vi "MAIN_8.1.vi"() -> ()   [LabVIEW 2015]
doc: "Use this template to build a producer/consumer design pattern with events to produce queue items. Use this design pattern instead of the User Interface Event Handler pattern for user interfaces when you want to execute code asynchronously in response to an event without slowing the user interface responsiveness."
uses:
  State_machine_enum.ctl
  display2.ctl
  User_buttons_enum.ctl
  <vilib>/Analysis/baseanly.llb/Mean (DBL).vi
  <vilib>/DAQmx/read.llb/DAQmx Read (Analog 2D DBL NChan NSamp).vi
  Global 1_diag.vi
  <vilib>/Waveform/WDTFileIO.llb/Export Waveforms To Spreadsheet File (1D).vi
  <vilib>/Utility/file.llb/Write To Spreadsheet File (DBL).vi
  <vilib>/DAQmx/create/channels.llb/DAQmx Create Channel (AI-Voltage-Basic).vi
  <vilib>/DAQmx/configure/timing.llb/DAQmx Timing (Sample Clock).vi
  <vilib>/DAQmx/miscellaneous.llb/DAQmx Fill In Error Info.vi
  <vilib>/express/express arith-compare/Formula/XNode/ExpressFormulaBlockNode.xnode
  <vilib>/Analysis/NI_AALBase.lvlib
  <resource>/objmgr/daqmx.rc
panel:
  out "2f Spectrum array":dbl[](array[numeric])
  out "x/y":dbl=0.002005684477504462
  in  "Motor Voltage (V) 2":dbl=1.0 min=0.0 max=9.0
  in  "Time Resolved":bool=TRUE
  in  "Start time":timestamp=timestamp(-9593251199.274853 s since 1904-01-01)
  in  "Timer Start":bool
  out "path":path=path "C:/Users/Adam/Desktop/Diag_Prog_v9/temp.txt"
  in  "Stabilization Time (s)":dbl min=0.0 max=2.0
  out "LD error array disc":dbl[](array[numeric])
  out "LD array disc":dbl[](array[numeric])
  out "result":bool=TRUE
  out "dt":dbl=0.001
  out "dLD_RMS":dbl=-0.0
  out "error out":errorcluster
  out "Unbalanced?":bool
  out "Signal Balance":bool
  out "DC Voltage (V) 2":dbl(knob)=0.000879695520089483 scale=0.0..10.0
  out "2f Frequency (Hz)":dbl(knob)=512.4961246512186 scale=0.0..150.0
  in  "Voltage Divider (10)":bool
  out "Actual Task":string="Processing signal"
  out "Motor Voltage (V)":dbl=1.0
  in  "Initial Voltage (V)":dbl=0.35 min=0.0 max=9.0
  in  "Final Voltage (V)":dbl=0.8 min=0.0 max=2.0
  in  "Voltage Step (V)":dbl=0.065 min=0.0 max=1000.0
  in  "Motor Stabilization Time (s)":dbl(knob)=10.0 step=0.001 scale=0.0..30.0
  out "Initial Voltage (V) 2":dbl=1.0 min=0.0 max=9.0
  in  "Final Voltage (V) 2":dbl=1.4 min=0.0 max=2.0
  in  "Voltage Step (V) 2":dbl=0.1 min=0.0 max=1000.0
  in  "Comment (sample no)":string
  in  "Stop Measurement":bool
  in  "Start Measurement Button":bool
  out "Measurement File":path=path "C:/Users/Adam/Desktop/Diag_Prog_v9/testt"
  in  "New File":bool
  out "Reset?":bool=TRUE
  out "Actual State":T1=enum."Process"
  in  "Tab Control":T2(tab)=enum."Options"
  out "Measured Points":T3 format="%0.3f"
  out "Ready?":bool
  out "Ready?":string="Ready?"
  out "Motor":bool=TRUE
  out "Motor":string="Motor: OK"
  out "Quick Status 5":string
  out "Down 2":bool
  out "Up 2":bool
  out "Oscilloscope 2":waveform(dbl)[](graph)=[{"t0"=timestamp(0 s since 1904-01-01), "dt"=0.002, "Y"=array[500 elements]}, {"t0"=timestamp(0 s since 1904-01-01), "dt"=0.002, "Y"=array[500 elements]}]
  out "Signal Balance":bool=TRUE
  out "Laser Noise":bool=TRUE
  out "Signal Balance":string="Signal Balance: OK"
  out "Laser Noise":string="Laser Noise: OK"
  in  "Run Quick Diagnostics":bool
  out "Laser Intensity":bool=TRUE
  out "Laser Intensity":string="Laser Intensity: OK"
  out "Delta":T3 format="%0.3f"
  out "Quick Diagnosis":string="?"
  out "Infected?":bool
  out "Detected Signal (mV/V)":T3 format="%0.3f"
  in  "Measure":bool
  out "Signal Spectrum (mVrms/Vdc) 2":cluster{"f0":dbl, "df":dbl, "magnitude":dbl[]}(graph)={"f0"=0.0, "df"=0.05, "magnitude"=[]}
  in  "QuickDiag":bool
  in  "Convert mld":bool
  in  "Convert parasiteno":bool
  in  "Convert parasitemia":bool
  in  "Convert cc":bool
  out "MLD (mV/V)":dbl=3.234067345901155 format="%#_3g"
  out "SA 1f (mv/V)":dbl=2.8989130211772483
  out "Lock_in (mV/V)":dbl
  out "dLock_in (mV/V)":dbl
  out "dMLD (mV/V)":dbl=1.4958145805121073 format="%#_3g"
  out "Phase (deg)":dbl=0.5117629371467104 format="%0.2f"
  out "Phase  dev (deg)":dbl=-1.4797919911802346 format="%0.2f"
  out "SA 2f (mv/V)":dbl=4.7886484733621755
  out "MLD Amplitude (mV/V)":cluster{dbl[], dbl[]}(graph)
  in  "dT/T (%)":dbl
  in  "Dilution":dbl=20.0
  in  "Undiluted cc.\n (ng/ml)":dbl
  in  "Undiluted \nParasitemia (%)":dbl format="%#_6f"
  in  "Parasites/ul\nof Blood":dbl
  in  "Convert dT":bool
  in  "MLD (mV/V)":dbl
  out "DC (V)":cluster{dbl[], dbl[]}(graph)
  out "MLD Phase":cluster{dbl[], dbl[]}(graph)
  out "Down":bool
  out "Up":bool
  out "2f Frequency (Hz)":T3=23.056300268096514 format="%0.3f"
  out "1f SA (mV/V)":T3=153.49895465158366 format="%0.3f"
  out "MLD Sim. LIA (mV/V)":T3=nan format="%0.3f"
  out "MLD SA (mV/V)":T3=37.38207236557522 format="%0.3f"
  in  "Start Scope":bool
  in  "Constant Motor Voltage":dbl=1.0 min=0.0 max=3.0
  in  "Refresh in (s)":i8=10
  in  "stop":bool
  in  "AC?":bool
  out "levelB":dbl=0.1 format="%#_2g"
  out "levelA":dbl format="%#_3g"
  in  "V/div B":dbl(knob)=0.2 scale=10.0..0.01 scale format="%#_3g"
  in  "level B":dbl(slide)=0.4 scale=-1.0..1.0 scale format="%#_3g"
  in  "level A":dbl(slide) scale=-1.0..1.0 scale format="%#_3g"
  in  "V/div A":dbl(knob)=0.05 scale=10.0..0.01 scale format="%#.3f"
  out "Oscilloscope":waveform(dbl)[](graph)=[{"t0"=timestamp(0 s since 1904-01-01), "dt"=0.0025, "Y"=array[375 elements]}, {"t0"=timestamp(0 s since 1904-01-01), "dt"=0.0025, "Y"=array[375 elements]}]
  in  "Sensitivity":T4(ring)
  in  "samples per channel":i32=1000
  in  "rate":dbl=1000.0 format="%0.2f"
  out "Spectrum (mVRMS/Vdc)":cluster{"f0":dbl, "df":dbl, "magnitude":dbl[]}(graph)={"f0"=0.0, "df"=1.0, "magnitude"=[1338.0484216778725, 891.4717650116102, 143.2192215595614, 172.79898091711885, 95.50453001628563, 113.23096269717587, 159.9728459536367, 142.17510842649094, 23.555096842939967, 172.4586840116519, 233.3391086271948, 153.49895465158366, 59.303017218056304, 51.41913744169332, 87.60985790792097, 89.15548748523767, 102.41083253503767, 116.69415211742178, 102.04780407888852, 98.07941394008398, 62.015801498942174, 57.365633541451224, 37.38207236557522, 140.01194138717574, 88.85968438008766, 51.8911573784031, 96.44625566359282, 102.80626369349147, 154.32416325374467, 152.72565881880075, 63.97627104136422, 44.061183722532256, 24.299532372372934, 66.51944362511281, 119.45636901763923, 79.60274206424093, 126.46507446936278, 115.56735495111872, 86.92439368676867, 42.47483057858276, 45.987972767001125, 82.38613913097223, 57.14235729256332, 24.715704736492583, 91.95786457200892, 229.45656360476565, 301.7932887816684, 181.94479488218664, 9.707170408716356, 79.16705422107816, 32.4671901662433, 34.994674897672475, 45.603676560961965, 81.17087782317107, 123.48392300390853, 125.53549820312338, 197.71297955832767, 51.56670220175255, 139.4897349387358, 136.00021553543283, 49.84751230386803, 106.388211919061, 128.21302631973177, 179.83380975700697, 238.686425101159, 204.64888147263136, 159.4400865495827, 88.9566203515302, 50.82386237011203, 47.10090178269198, 31.249556983451996, 155.07366739734923, 197.20488460315576, 181.86491698592144, 122.60135896300172, 15.723508058553668, 47.32988919426525, 91.09235604990127, 70.08764782926058, 71.11042986773145, 167.58334514547386, 157.0684001711449, 85.4088975978964, 165.68125229281705, 108.34787076535925, 58.32465184772515, 102.85811162079386, 88.031264754637, 35.99088343784742, 74.99228300753498, 59.59436041355427, 109.74543517855098, 239.92689639368845, 195.22681808589817, 153.93792803433803, 171.35120542643082, 103.04216715301814, 144.22424620891795, 33.236928017526, 33.6474288996255, 71.18496484217899, 175.10446025244616, 221.24997378317522, 114.75466832528755, 52.3833439055373, 114.90211538243959, 94.87498722211751, 82.82924122532899, 124.12586199482064, 107.6258638888207, 78.5024563400891, 92.06245924719637, 16.228987466475928, 84.84217000760313, 88.76503911599063, 114.25618103440272, 155.27289903749065, 116.20062823456668, 61.96139303164934, 214.19314697712042, 248.12058486418763, 215.9112937618697, 145.04293815290015, 142.16464369485132, 169.7377761460246, 83.55657324380019, 74.4879617799582, 39.81106304135121, 152.2410798694005, 176.4879867987291, 110.01229615691923, 89.83888006443468, 195.69702436303007, 166.19892376632072, 55.02836867851484, 113.06515146784245, 221.3685360221306, 181.10055208661387, 262.0371181638539, 185.73443857709046, 93.90961856721144, 84.54783744027858, 24.449872475327695, 95.3789149136639, 140.24246950513043, 143.73337464437884, 33.58378655631947, 62.839362697344995, 57.47449635929643, 139.96968907631262, 167.0231838520772, 135.6723918020847, 124.14523269479409, 111.37946391963057, 195.70470757666732, 192.9947832776428, 93.91006382282066, 121.56931305302999, 113.63589006917633, 42.92804035457153, 141.48803985115433, 165.5507518379778, 121.34962379960878, 143.04362518480343, 22.72432951654588, 183.17549468524615, 152.95042171438013, 195.3079831947777, 131.83171839040367, 30.49881104219535, 8.46043248589554, 141.40803256070282, 223.72992955634092, 132.30059550265176, 54.60897309407436, 84.56504745319246, 125.72411835874722, 194.72474433717994, 126.94182365881618, 27.456941187399302, 114.85067679816903, 138.3914927403539, 237.22038521157256, 172.58040690453, 178.93819766022105, 171.11586449112946, 66.32529189912087, 175.61268977844438, 179.0727535154661, 223.71442469320746, 230.52161416220554, 181.0440521026372, 72.70233235363926, 157.99312186800248, 143.29067791998708, 138.45794114882568, 122.15383561979628, 55.90884824057415, 43.2895289444191, 25.99180252149831]}
  out "MLD LIA (mV/V)":dbl=0.0123978
  out "Lockin_freq":dbl=9.4676
  out "DC Voltage (V)":T3=0.000879695520089483 format="%0.3f"
  out "Time Domain Signal":cluster{"xi used":dbl[], "yi":dbl[]}[](graph)
  out "Signal Spectrum (mVrms/Vdc)":cluster{"f0":dbl, "df":dbl, "magnitude":dbl[]}[](graph)
  out "1f 2f Spectral Peaks":T5={"1f (Hz)"=256.112805640282, "U1f (mV/V)"=2.8989130211772483, "2f (Hz)"=512.375618780939, "U2f (mV/V)"=4.7886484733621755}
  out "LockIN Theta (cont/disc)":waveform(dbl)(graph)={"t0"=timestamp(0 s since 1904-01-01), "dt"=0.002, "Y"=[]}
  out "LockIN R (cont/disc)":waveform(dbl)(graph)={"t0"=timestamp(0 s since 1904-01-01), "dt"=0.002, "Y"=[]}
  in  "Pike Removal (StDev)":dbl=3.0
  in  "Lock-in Time (s)":dbl=10.0
  in  "dt (s)":dbl=0.0002
  in  "Resolution (s)":dbl=0.0001
  in  "Averaging time (s)":dbl=1.0 format="%0.2p"
  in  "Cutoff Frequency (Hz)":dbl=500.0
  in  "Rate":dbl=5000.0 caption="Sample Rate (Hz)" format="%0.2f"
  in  "Samples per Channel":i32=100000
  out "Minimum Value":dbl=-1.0 caption="LD min Value (V)" format="%0.2f"
  out "Maximum Value":dbl=1.0 caption="LD max Value (V)" format="%0.2f"
  in  "DC # samples":i32=100
  in  "DC Sampling Rate (Hz)":dbl=100.0
  in  "Dc min":dbl format="%0.2f"
  in  "Dc max":dbl=10.0 format="%0.2f"
  in  "Reference Signal":tag="Dev1/ai3"
  in  "LD Signal":tag="Dev1/ai0" caption="LD Channel"
  in  "DC Voltage DAQ":tag="Dev1/ai1"
  in  "Motor Channel":tag="Dev1/ao1"
  in  "Lock-in-Amplifier VISA":refnum<visa-resource-name>="GPIB0::3::INSTR"
  in  "Second Harmonic":bool
  in  "Lock In":bool
  in  "Continous Lock-in":bool=TRUE
  out "Dc standard deviation":dbl=0.002551891780639937 format="%0.2f"
  out "Dc mean":dbl=0.000879695520089483 format="%0.2f"
  out "dPhase array":dbl[](array[numeric])=[0.7103181848590662, 0.7091849884099535, 0.5117629371467104]
  out "Phase array":dbl[](array[numeric])=[2.6241958943190986, 1.203559524600966, nan, 1.2024263281518537, -0.21594364866805338, nan, -1.4797919911802346]
  out "LD array":dbl[](array[numeric])=[0.8882278113428617, 1.3288564379056984, 3.234067345901155]
  out "Frequency array":dbl[](array[numeric])=[811.3544417222341, 812.123069024086, 812.8874794085821]
  out "LD error array":dbl[](array[numeric])=[0.357199186111431, 0.6995380180896104, 1.4958145805121073]
  out "First?":bool
  out "Stopped":bool
  out "Last Step?":bool
  in  "EXIT":bool
  # "Measurement Settings"
  # "Motor Setup"
  # "OFF"
  # "ON"
  # "Setup"
  # "Status:"
  # "Measurement"
  # "mV/V"
  # "±"
  # "Detected Magneto-Optical Signal:"
  # "Quick Diagnosis Report:"
  # "Measured points:"
  # "Actual Datapoint Values"
  # "Convert quantities"
  # "Physical channels"
  # "Signal Processing Settings"
  # "DC Acquisition Settings"
  # "LD Acquisition Settings"
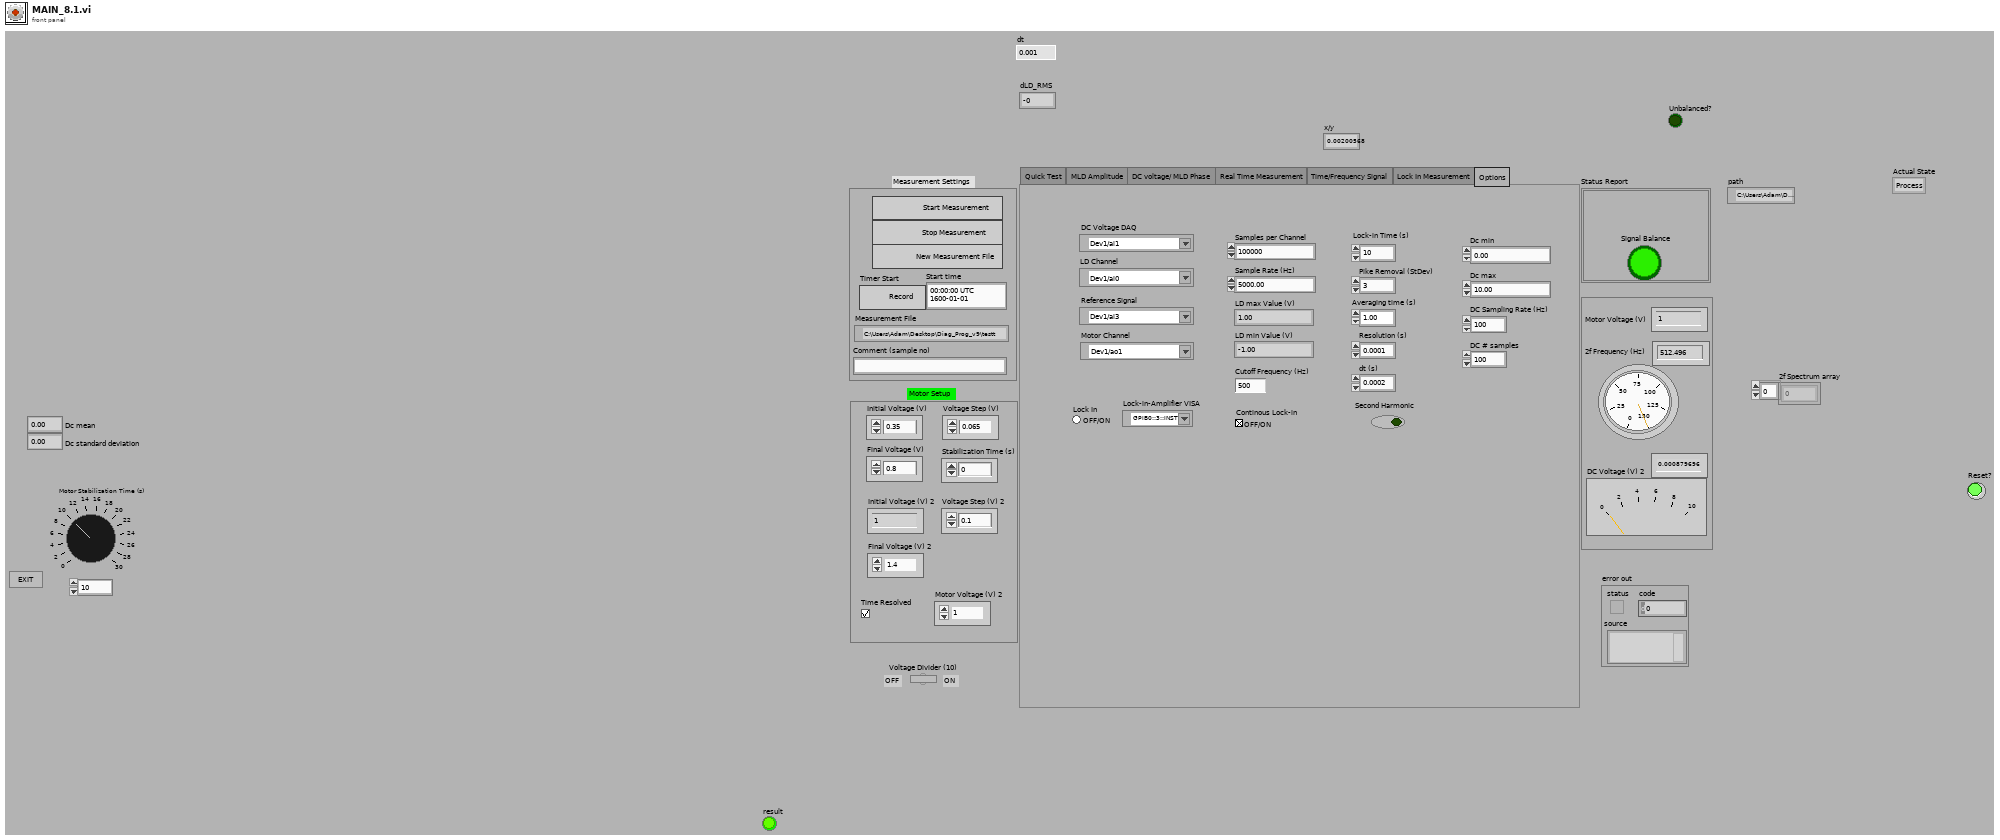
[diagram p1: front panel]
types:
  T1 = typedef "State_machine_enum.ctl" = enum16{"SetMotor", "Stabilize", "Measure", "Process", "Save", "Finished"}
  T2 = enum32{"Quick Test", "MLD Amplitude", "DC voltage/ MLD Phase", "Real Time Measurement", "Time/Frequency Signal", "Lock In Measurement", "Options"}
  T3 = typedef "display2.ctl" = dbl
  T4 = enum16{"-1V..1V", "-1.25V..1.25V", "-2V..2V", "-2.5V..2.5V", "-4V..4V", "-5V..5V", "-10V..10V"}
  T5 = cluster{"1f (Hz)":dbl, "U1f (mV/V)":dbl, "2f (Hz)":dbl, "U2f (mV/V)":dbl}
  T6 = typedef "User_buttons_enum.ctl" = enum16{"start", "stop", "exit", "New", "Scope", "Continue"}
  T7 = enum16{"open", "replace", "create", "open or create", "replace or create", "replace or create with confirmation"}
  T8 = enum8{"Enabled", "Disabled", "Disabled and Grayed Out"}
  T9 = enum16{"Left Button", "Center Button", "Right Button", "Window Close"}
  T10 = cluster{dbl, "1f Ampl (Vrms/Vdc)":dbl, dbl, "2f Ampl (Vrms/Vdc)":dbl}
  T11 = cluster{"MLD":dbl, "dMLD":dbl, "Phase":dbl, "dPhase":dbl}
  T12 = cluster{"Frequency array":dbl[], "LD array":dbl[]}
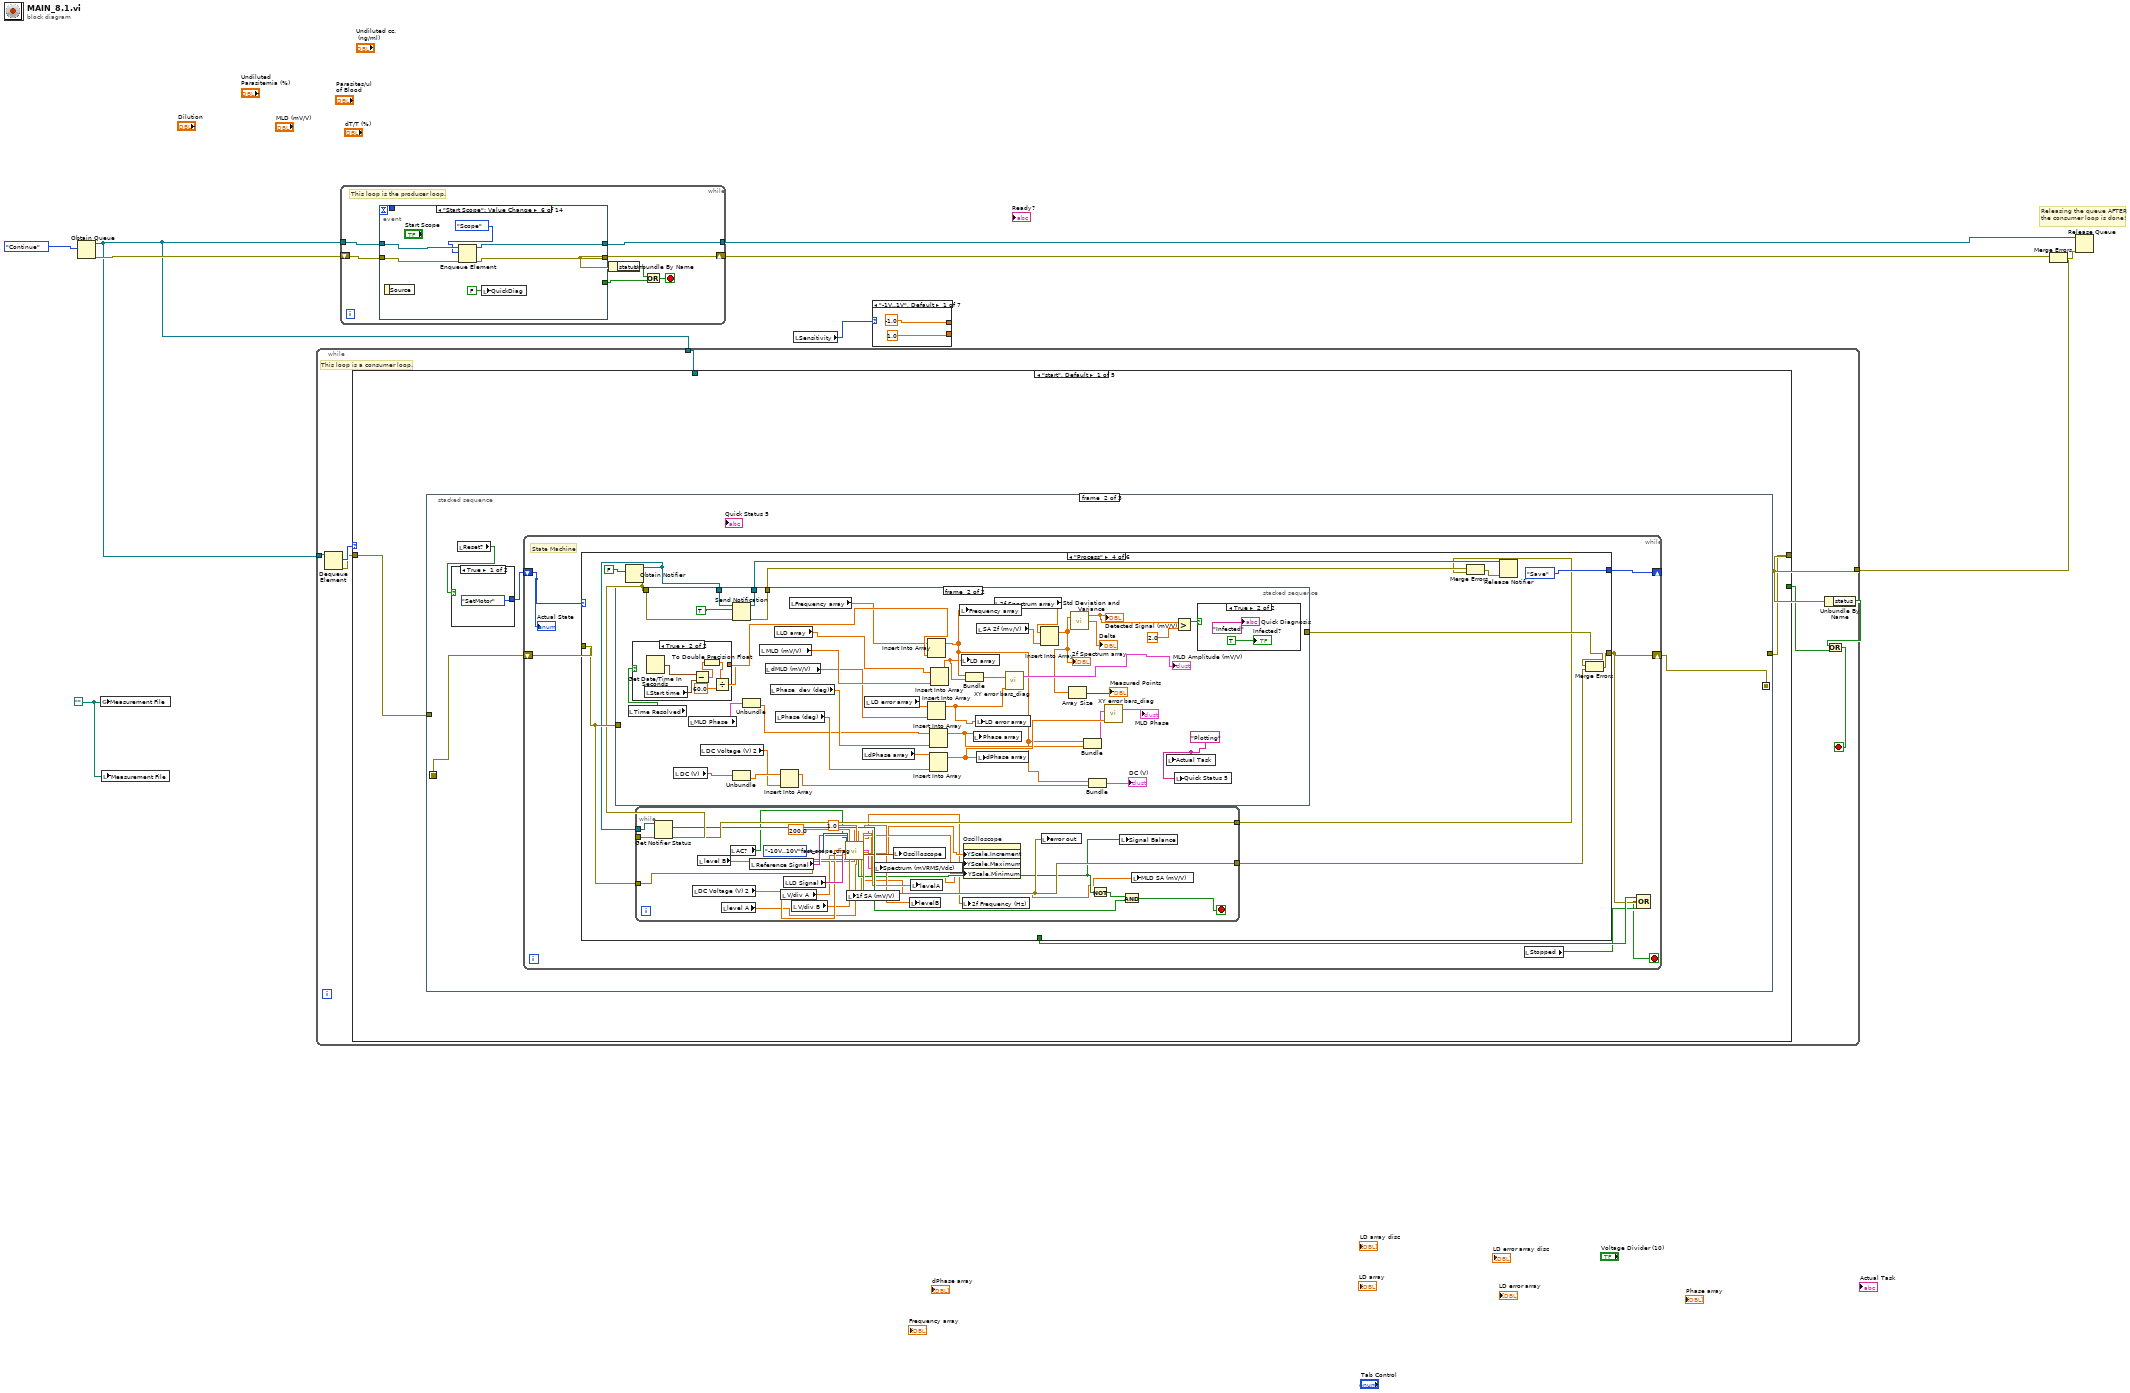
[diagram p0: block diagram]
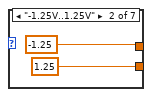
[diagram p2: hidden frame]
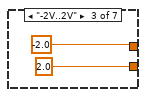
[diagram p3: hidden frame]
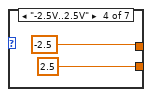
[diagram p4: hidden frame]
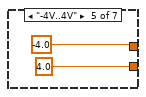
[diagram p5: hidden frame]
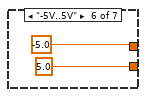
[diagram p6: hidden frame]
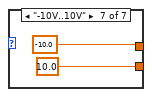
[diagram p7: hidden frame]
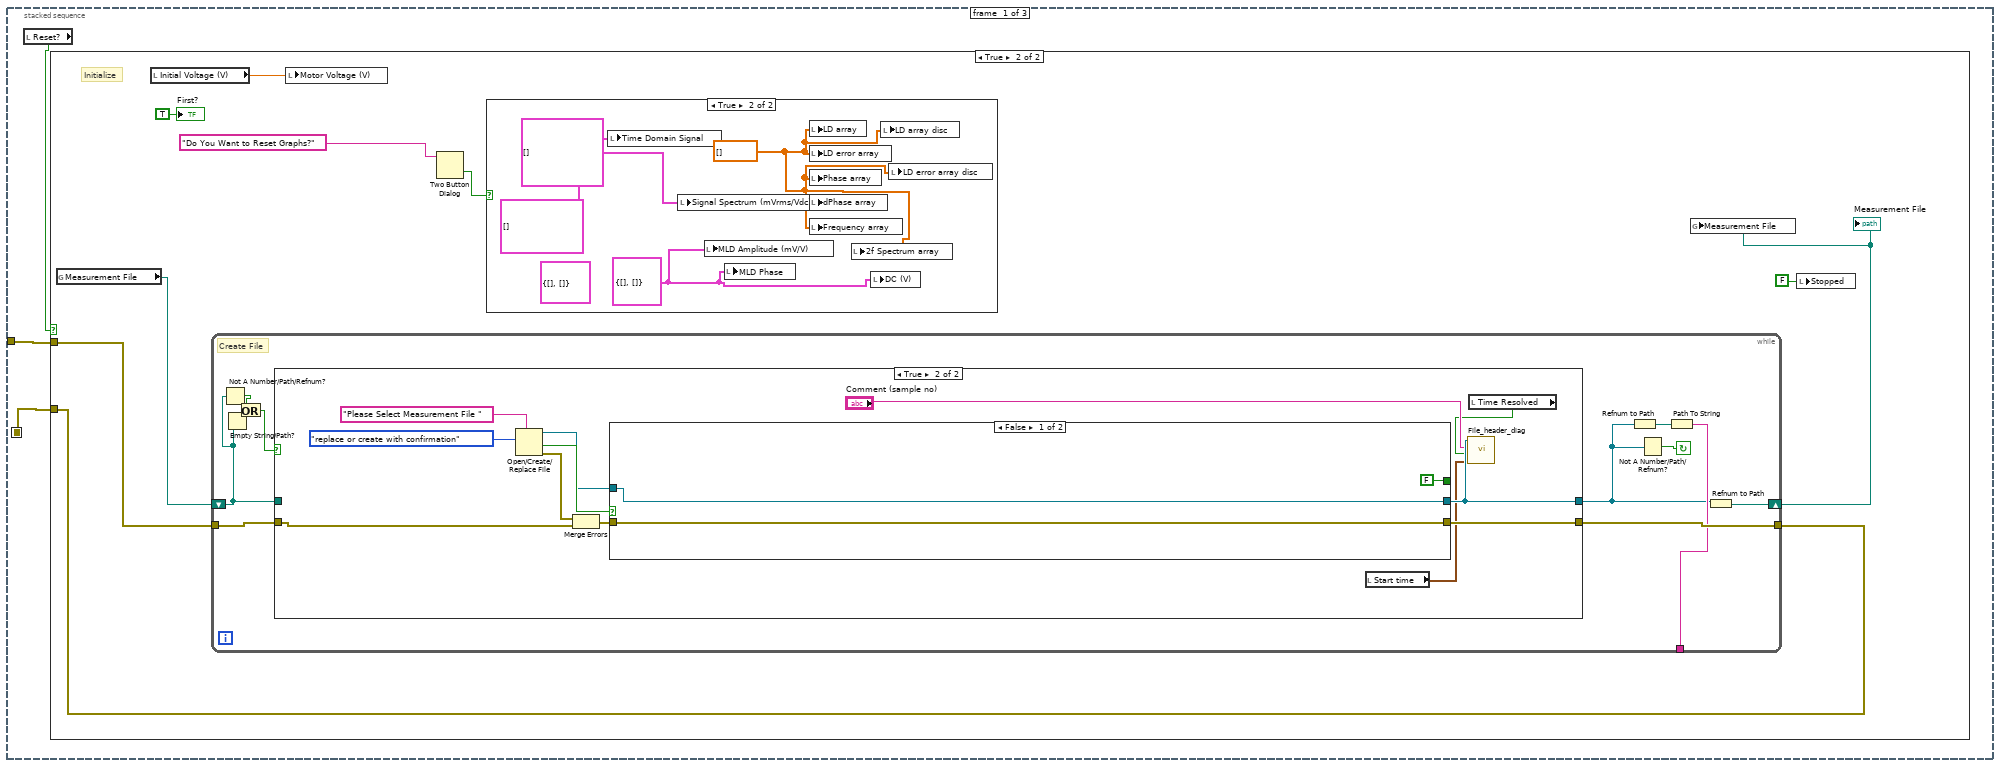
[diagram p8: hidden frame]
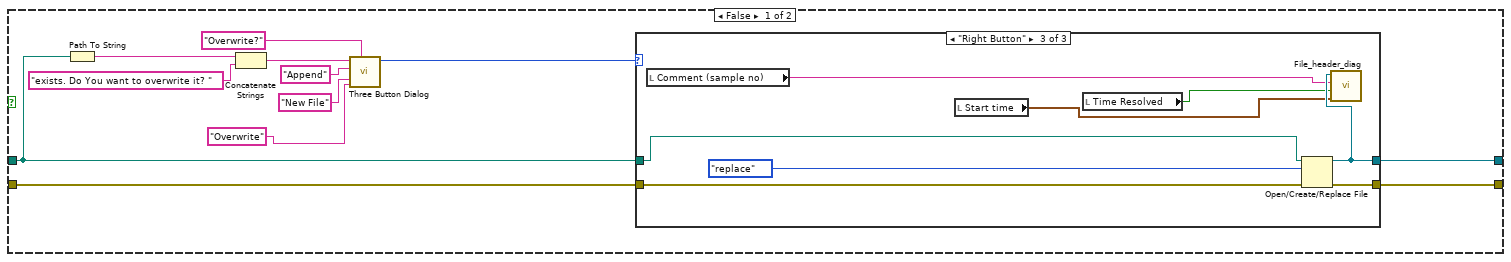
[diagram p10: hidden frame]
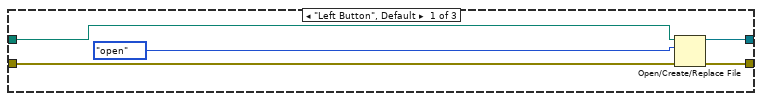
[diagram p11: hidden frame]
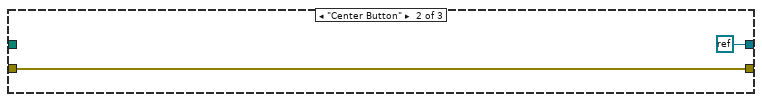
[diagram p12: hidden frame]
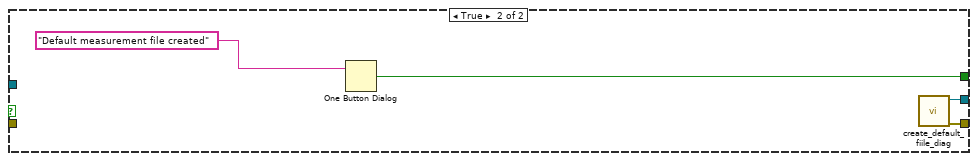
[diagram p13: hidden frame]
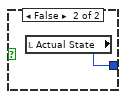
[diagram p15: hidden frame]
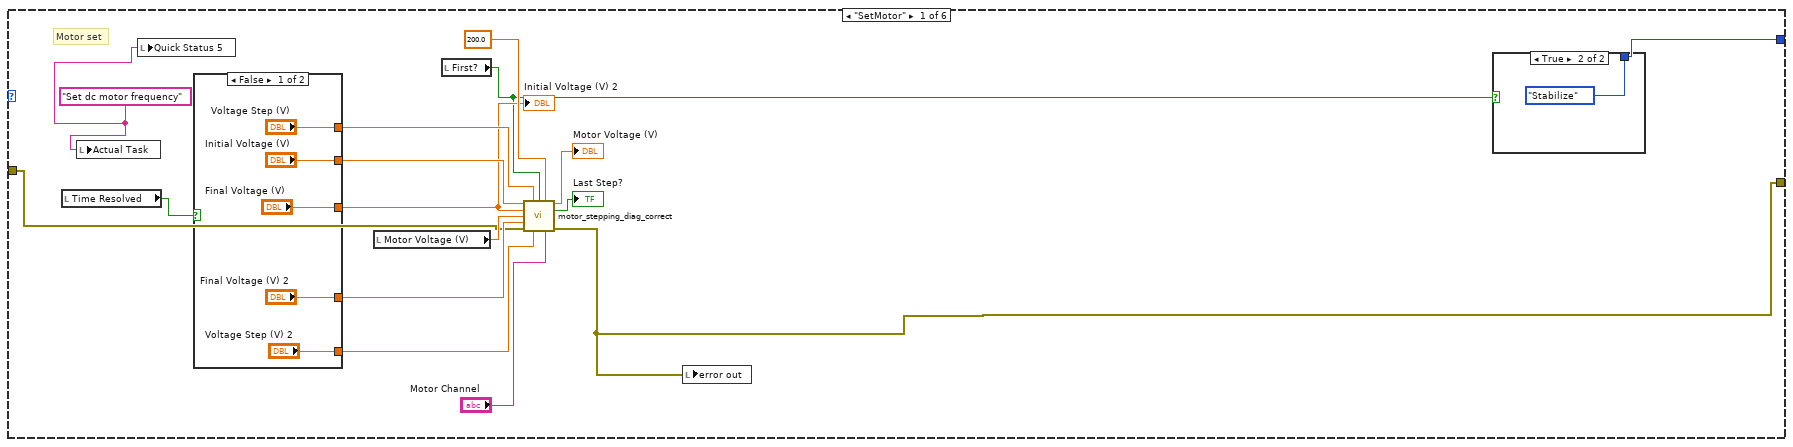
[diagram p16: hidden frame]
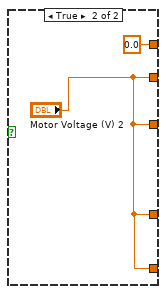
[diagram p17: hidden frame]
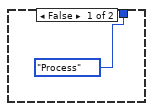
[diagram p18: hidden frame]
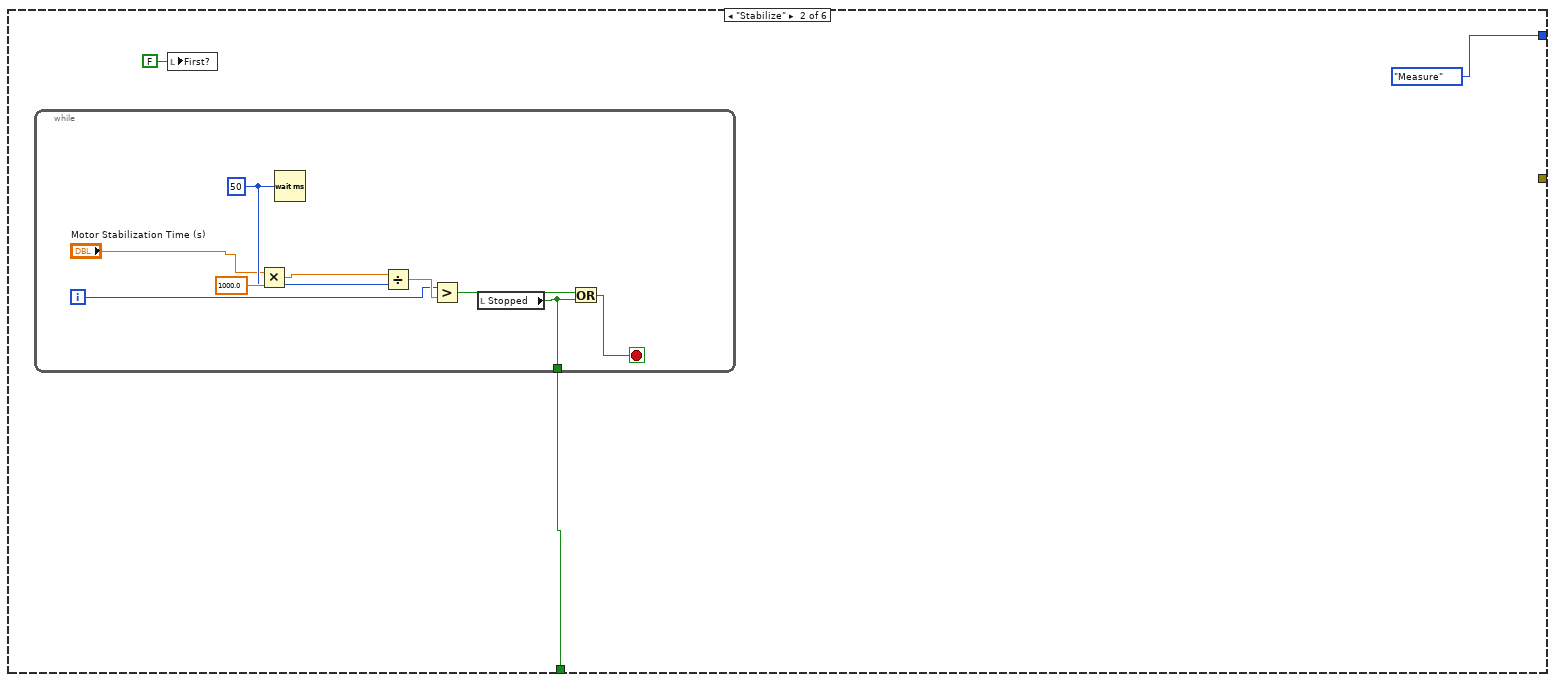
[diagram p19: hidden frame]
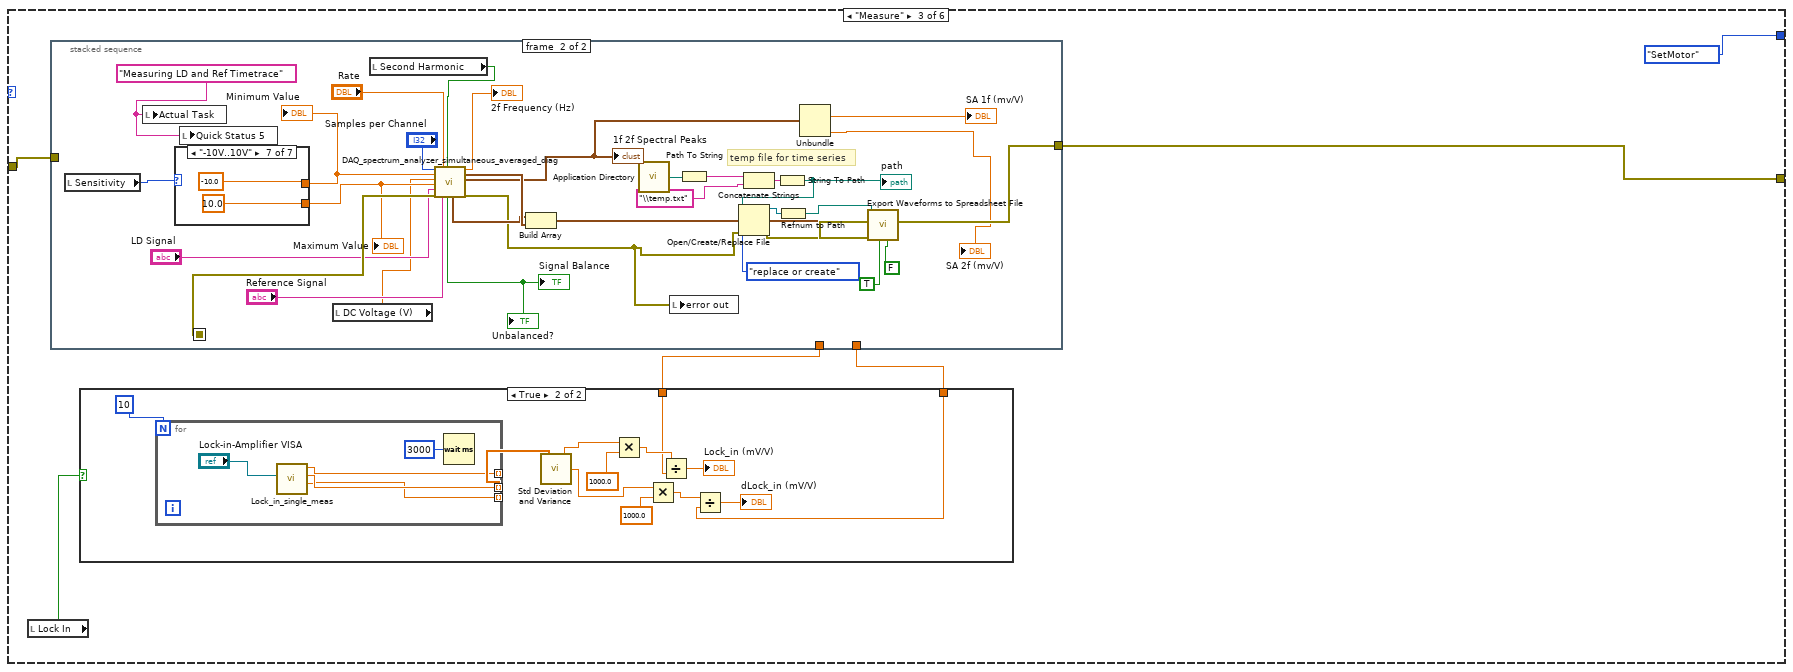
[diagram p20: hidden frame]
diagram:
  w3 = path ""
  # "Releasing the queue AFTER\nthe consumer loop is done!"
  n1 = Obtain Queue(element data type=User_buttons_enum."Continue") -> (queue out=w2:refnum<queue>, error out=w9:errorcluster)  [unwired: 4 in, 1 out]
  n2 = global write "Global 1_diag.vi" "Measurement File"(w3) -> ()
  n3 = local write "Measurement File"(w3) -> ()
  n4 = while {
    tunnel: w2 -> [w17]
    tunnel: [w14] -> w5
    tunnel: w2 -> [w10]
    stop <- w11 stop-if-true
    # "This loop is a consumer loop."
    n5 = Dequeue Element(queue=w17) -> (element=w16:T6, error out=w15:errorcluster)  [unwired: 2 in, 2 out]
    n6 = case shown="\"start\", Default" w16 {
      tunnel: [_ _ TRUE _ _] -> w12
      tunnel: w15 -> [w19 w418 w480 w484 w493]
      tunnel: [w18 w417 w480 w483 w499] -> w14
      tunnel: w10 -> [_ w416 _ _ w485]
      frame "start", Default {
        n7 = stacked-sequence {
          seq-local: [w21 _ _] -> [_ w97 _]
          seq-local: [_ w96 _] -> [_ _ w403]
          tunnel: w19 -> [w22 _ w401]
          tunnel: [_ _ w400] -> w18
          frame #0 {
            n8 = local read "Reset?"() -> (w20:bool)
            n9 = case shown="True" w20 {
              tunnel: w22 -> [w23 w27]
              tunnel: [w23 w25] -> w21
              frame False {
              }
              frame True {
                # "Initialize"
                n10 = global read "Global 1_diag.vi" "Measurement File"() -> (w26:path)
                n11 = local read "Initial Voltage (V)"() -> (w30:dbl)
                n12 = while {
                  tunnel: [w43] -> w25
                  tunnel: w27 -> [w42]
                  shift-right: [w37] -> w24
                  shift-left: w26 -> [w36]
                  tunnel: [w39] -> _
                  stop <- w41 continue-if-true
                  # "Create File"
                  n13 = Not A Number/Path/Refnum?(number/path/refnum=w36) -> (NaN/Path/Refnum?=w35:bool)
                  n14 = Empty String/Path?(string/path=w36) -> (empty?=w34:bool)
                  n15 = Or(x=w35, y=w34) -> (x .or. y?=w33:bool)
                  n16 = case shown="True" w33 {
                    tunnel: [w50 w75] -> w38
                    tunnel: [w49 w74] -> w43
                    tunnel: w42 -> [w48 w76]
                    tunnel: w36 -> [w44 _]
                    frame False {
                      n17 = Path To String(path=w44) -> (string=w47:string)
                      n18 = Concatenate Strings(w47, "exists. Do You want to overwrite it? " ("message")) -> (w45:string)
                      n19 = call <vilib>:"Three Button Dialog.vi"("Window Title (\"\")"="Overwrite?" ("Window Title (\"\")"), "Right Button Text (\"Cancel\")"="Overwrite" ("Right Button Text (\"Cancel\")"), "Center Button Text (\"No\")"="New File" ("Center Button Text (\"No\")"), "Left Button Text (\"Yes\")"="Append" ("Left Button Text (\"Yes\")"), "message"=w45) -> ("Which Button?"=w51:T9)  [unwired: 6 in]
                      n20 = case shown="\"Right Button\"" w51 {
                        tunnel: w44 -> [w56 _ w66]
                        tunnel: [w57 refnum<k0> refnum w67] -> w50
                        tunnel: [w59 w61 w69] -> w49
                        tunnel: w48 -> [w58 w61 w68]
                        frame "Left Button", Default {
                          n21 = Open/Create/Replace File(file path (use dialog)=w56, error in=w58, operation (0:open)=T7."open") -> (refnum out=w57:refnum<file>, error out=w59:errorcluster)  [unwired: 3 in, 1 out]
                        }
                        frame "Center Button" {
                        }
                        frame "Right Button" {
                          n22 = local read "Comment (sample no)"() -> (w65:string)
                          n23 = local read "Start time"() -> (w63:timestamp)
                          n24 = local read "Time Resolved"() -> (w64:bool)
                          n25 = Open/Create/Replace File(file path (use dialog)=w66, error in=w68, operation (0:open)=T7."replace") -> (refnum out=w67:refnum<file>, error out=w69:errorcluster)  [unwired: 3 in, 1 out]
                          n26 = call "File_header_diag.vi"("Preparation time"=w63, "Time resolved?"=w64, "Comment"=w65, "Byte Stream File in"=w67) -> ()  [unwired: 8 in]
                        }
                      }
                    }
                    frame True {
                      n27 = Open/Create/Replace File(prompt="Please Select Measurement File ", operation (0:open)=T7."replace or create with confirmation") -> (refnum out=w79:refnum<file>, cancelled=w80:bool, error out=w78:errorcluster)  [unwired: 4 in]
                      n28 = Merge Errors(w78, w76) -> (w77:errorcluster)
                      n29 = case shown="False" w80 {
                        tunnel: w79 -> [w85 _]
                        tunnel: [w85 w86] -> w75
                        tunnel: [w84 w88] -> w74
                        tunnel: w77 -> [w84 _]
                        tunnel: [FALSE ("true") w87] -> _
                        frame False {
                        }
                        frame True {
                          n30 = One Button Dialog(message="Default measurement file created") -> (true=w87:bool)  [unwired: 1 in]
                          n31 = call "create_default_fiile_diag.vi"() -> ("error out"=w88:errorcluster, "Byte Stream File out"=w86:refnum<file>)  [unwired: 10 in]
                        }
                      }
                      n32 = local read "Start time"() -> (w71:timestamp)
                      n33 = local read "Time Resolved"() -> (w72:bool)
                      n34 = call "File_header_diag.vi"("Preparation time"=w71, "Time resolved?"=w72, "Comment"="Comment (sample no)", "Byte Stream File in"=w75) -> ()  [unwired: 8 in]
                    }
                  }
                  n35 = Refnum to Path(1:w38) -> (0:w40:path)
                  n36 = Not A Number/Path/Refnum?(number/path/refnum=w38) -> (NaN/Path/Refnum?=w41:bool)
                  n37 = Path To String(path=w40) -> (string=w39:string)
                  n38 = Refnum to Path(1:w38) -> (0:w37:path)
                }
                "Measurement File" <- w24
                n39 = local write "Motor Voltage (V)"(w30) -> ()
                n40 = Two Button Dialog(message="Do You Want to Reset Graphs?") -> (T button?=w28:bool)  [unwired: 2 in]
                n41 = case shown="True" w28 {
                  frame False {
                  }
                  frame True {
                    w91 = cluster{dbl[], dbl[]} {[], []} ("MLD Amplitude (mV/V)")
                    (unwired) cluster{"magnitude":dbl[], "magnitude 2":dbl[]} {"magnitude"=[], "magnitude 2"=[]} ("MLD Amplitude")
                    w90 = dbl[] []
                    n42 = local write "Time Domain Signal"(cluster{dbl[], dbl[]}[] [] ("Integral")) -> ()
                    n43 = local write "Signal Spectrum (mVrms/Vdc)"(cluster{"f0":dbl, "df":dbl, dbl[]}[] [] ("Signal Spectrum")) -> ()
                    n44 = local write "MLD Amplitude (mV/V)"(w91) -> ()
                    n45 = local write "MLD Phase"(w91) -> ()
                    n46 = local write "LD array"(w90) -> ()
                    n47 = local write "LD error array"(w90) -> ()
                    n48 = local write "Phase array"(w90) -> ()
                    n49 = local write "dPhase array"(w90) -> ()
                    n50 = local write "Frequency array"(w90) -> ()
                    n51 = local write "2f Spectrum array"(w90) -> ()
                    n52 = local write "DC (V)"(w91) -> ()
                    n53 = local write "LD array disc"(w90) -> ()
                    n54 = local write "LD error array disc"(w90) -> ()
                  }
                }
                n55 = global write "Global 1_diag.vi" "Measurement File"(w24) -> ()
                n56 = local write "Stopped"(FALSE ("Stopped")) -> ()
                "First?" <- TRUE ("First?")
              }
            }
          }
          frame #1 {
            n57 = local read "Reset?"() -> (w94:bool)
            n58 = case shown="True" w94 {
              tunnel: [State_machine_enum."SetMotor" w99] -> w95
              frame True {
              }
              frame False {
                n59 = local read "Actual State"() -> (w99:T1)
              }
            }
            n60 = while {
              shift-right: [w100] -> _
              shift-left: w95 -> [w106]
              shift-right: [w104] -> w96
              shift-left: w97 -> [w101]
              stop <- w102 stop-if-true
              # "State Machine"
              n61 = case shown="\"Process\"" w106 {
                tunnel: [w108 _ w149 w233 w388 _] -> w104
                tunnel: [_ w134 _ _ _ w399] -> w105
                tunnel: w101 -> [w117 _ w148 w231 w388 _]
                tunnel: [w122 State_machine_enum."Measure" State_machine_enum."SetMotor" State_machine_enum."Save" w387 State_machine_enum."SetMotor"] -> w100
                frame "SetMotor" {
                  w107 = "Set dc motor frequency" ("Actual Task")
                  # "Motor set"
                  n62 = local read "Time Resolved"() -> (w109:bool)
                  n63 = local write "Actual Task"(w107) -> ()
                  n64 = local write "Quick Status 5"(w107) -> ()
                  n65 = case shown="False" w109 {
                    tunnel: ["Initial Voltage (V)" "Motor Voltage (V) 2"] -> w121
                    tunnel: ["Final Voltage (V) 2" "Motor Voltage (V) 2"] -> w118
                    tunnel: ["Voltage Step (V)" 0.0 ("Voltage Step (V)")] -> w116
                    tunnel: ["Voltage Step (V) 2" "Motor Voltage (V) 2"] -> w115
                    tunnel: ["Final Voltage (V)" "Motor Voltage (V) 2"] -> w111
                    frame False {
                    }
                    frame True {
                    }
                  }
                  "Initial Voltage (V) 2" <- w111
                  n66 = local read "Motor Voltage (V)"() -> (w119:dbl)
                  n67 = local read "First?"() -> (w110:bool)
                  n68 = call "motor_stepping_diag_correct.vi"("Initial Voltage (V)"=w121, "Voltage Step (V)"=w116, "First?"=w110, "Steps"=200.0, "Final Voltage (V)"=w111, "Actual Voltage (V)  in"=w119, "Final Voltage (V) 2"=w118, "error in (no error)"=w117, "Voltage Step2"=w115, "Physical Channel"="Motor Channel") -> ("Actual Voltage (V)"=→"Motor Voltage (V)":dbl, "Boolean"=→"Last Step?":bool, "error out"=w108:errorcluster)  [unwired: 3 in]
                  n69 = local write "error out"(w108) -> ()
                  n70 = case shown="True" w110 {
                    tunnel: [State_machine_enum."Process" State_machine_enum."Stabilize"] -> w122
                    frame False {
                    }
                    frame True {
                    }
                  }
                }
                frame "Stabilize" {
                  n71 = while {
                    tunnel: [w135] -> w134
                    i -> [w136]
                    stop <- w138 stop-if-true
                    w141 = u32 50 ("milliseconds to wait")
                    n72 = Multiply(x="Motor Stabilization Time (s)", y=1000.0) -> (x*y=w143:dbl)
                    n73 = Wait (ms)(milliseconds to wait=w141) -> ()  [unwired: 1 out]
                    n74 = Divide(x=w143, y=w141) -> (x/y=w140:dbl)
                    n75 = Greater?(x=w136, y=w140) -> (0:w139:bool)
                    n76 = local read "Stopped"() -> (w135:bool)
                    n77 = Or(x=w139, y=w135) -> (x .or. y?=w138:bool)
                  }
                  n78 = local write "First?"(FALSE ("First?")) -> ()
                }
                frame "Measure" {
                  n79 = local read "Lock In"() -> (w144:bool)
                  n80 = stacked-sequence {
                    seq-local: [w173 _] -> [_ w210]
                    tunnel: [_ w209] -> w149
                    tunnel: w148 -> [w169 _]
                    tunnel: [w168 _] -> w147
                    tunnel: [w168 _] -> w146
                    frame #0 {
                      w167 = "Measuring DC Voltage" ("Actual Task")
                      n81 = local write "Actual Task"(w167) -> ()
                      n82 = local write "Quick Status 5"(w167) -> ()
                      n83 = call "manualDAQ_diag.vi"("minimum value"="Dc min", "Rate"="DC Sampling Rate (Hz)", "error in (no error)"=w169, "Samples per Channel"="DC # samples", "maximum value"="Dc max", "physical channels"="DC Voltage DAQ") -> ("error out"=w173:errorcluster, "output waveform"=w175:waveform(dbl))  [unwired: 4 in]
                      "error out" <- w173
                      n84 = Unbundle By Name(w175) -> ("Y"=w176:dbl[])
                      n85 = call <vilib>:"Std Deviation and Variance.vi"("X"=w176) -> ("mean"=w168:dbl, "standard deviation"=→"Dc standard deviation":dbl)  [unwired: 1 in, 1 out]
                      "DC Voltage (V) 2" <- w168
                      "Dc mean" <- w168
                      n86 = local write "DC Voltage (V)"(w168) -> ()
                    }
                    frame #1 {
                      w179 = "Measuring LD and Ref Timetrace" ("Actual Task")
                      # "temp file for time series"
                      n87 = local read "Sensitivity"() -> (w196:T4)
                      n88 = local write "Actual Task"(w179) -> ()
                      n89 = case shown="\"-10V..10V\"" w196 {
                        tunnel: [-1.0 ("maximum value") -1.25 ("maximum value") -2.0 ("maximum value") -2.5 ("maximum value") -4.0 ("maximum value") -5.0 ("maximum value") -10.0 ("maximum value")] -> w195
                        tunnel: [1.0 ("maximum value") 1.25 ("maximum value") 2.0 ("maximum value") 2.5 ("maximum value") 4.0 ("maximum value") 5.0 ("maximum value") 10.0 ("maximum value")] -> w194
                        frame "-1V..1V", Default {
                        }
                        frame "-1.25V..1.25V" {
                        }
                        frame "-2V..2V" {
                        }
                        frame "-2.5V..2.5V" {
                        }
                        frame "-4V..4V" {
                        }
                        frame "-5V..5V" {
                        }
                        frame "-10V..10V" {
                        }
                      }
                      "Maximum Value" <- w194
                      "Minimum Value" <- w195
                      n90 = local write "Quick Status 5"(w179) -> ()
                      n91 = local read "DC Voltage (V)"() -> (w193:T3)
                      n92 = local read "Second Harmonic"() -> (w180:bool)
                      n93 = call "DAQ_spectrum_analyzer_simultaneous_averaged_diag.vi"("Samples per Channel"="Samples per Channel", "minimum value"=w195, "DC voltage (V)"=w193, "maximum value"=w194, "LD channel"="LD Signal", "Error In"=w210, "Rate"="Rate", "Ref channel"="Reference Signal", "Second"=w180) -> ("Unbalanced?"=→"Signal Balance" →"Unbalanced?":bool, "raw signal waveform"=w199:waveform(dbl), "Calculated frequency"=→"2f Frequency (Hz)":dbl, "Reference Timetrace"=w200:waveform(dbl), "1f 2f"=w198:T10, "error out"=w185:errorcluster)  [unwired: 5 out]
                      "1f 2f Spectral Peaks" <- w198
                      n94 = Build Array(w199, w200) -> (w202:waveform(dbl)[])
                      n95 = call <vilib>:"Application Directory.vi"() -> ("Application Directory"=w190:path)
                      n96 = local write "error out"(w185) -> ()
                      n97 = Path To String(path=w190) -> (string=w189:string)
                      n98 = Concatenate Strings(w189, "\\temp.txt" ("element")) -> (w187:string)
                      n99 = String To Path(string=w187) -> (path=w183:path)
                      "path" <- w183
                      n100 = Open/Create/Replace File(file path (use dialog)=w183, error in=w185, operation (0:open)=T7."replace or create") -> (refnum out=w182:refnum<file>, error out=w184:errorcluster)  [unwired: 3 in, 1 out]
                      n101 = Refnum to Path(1:w182) -> (0:w181:path)
                      n102 = Unbundle(w198) -> ("1f Ampl (Vrms/Vdc)"=→"SA 1f (mv/V)":dbl, "2f Ampl (Vrms/Vdc)"=→"SA 2f (mv/V)":dbl)  [unwired: 2 out]
                      n103 = call-poly <vilib>:"Export Waveforms to Spreadsheet File.vi"("header? (write header:T)"=FALSE, "append to file? (new file:F)"=TRUE ("header? (write header:T)"), "error in (no error)"=w184, "waveforms"=w202, "file path (dialog if empty)"=w181) -> ("error out"=w209:errorcluster)  [unwired: 5 in, 1 out]
                    }
                  }
                  n104 = case shown="True" w144 {
                    tunnel: w147 -> [_ w156]
                    tunnel: w146 -> [_ w152]
                    frame False {
                    }
                    frame True {
                      n105 = for {
                        N: 10 -> [_]
                        tunnel: [w164] -> _ mode=indexing
                        tunnel: [w163] -> w160 mode=indexing
                        tunnel: [w162] -> _ mode=indexing
                        n106 = call "Lock_in_single_meas.vi"("Lock-in-Amplifier VISA"="Lock-in-Amplifier VISA") -> ("Lockin_phas"=w162:dbl, "Lockin_ampl"=w163:dbl, "Freq"=w164:dbl)  [unwired: 7 in, 1 out]
                        n107 = Wait (ms)(milliseconds to wait=u32 3000) -> ()  [unwired: 1 out]
                      }
                      n108 = call <vilib>:"Std Deviation and Variance.vi"("X"=w160) -> ("mean"=w159:dbl, "standard deviation"=w153:dbl)  [unwired: 1 in, 1 out]
                      n109 = Multiply(x=w159, y=1000.0) -> (x*y=w157:dbl)
                      n110 = Multiply(x=w153, y=1000.0) -> (x*y=w155:dbl)
                      n111 = Divide(x=w157, y=w156) -> (x/y=→"Lock_in (mV/V)":dbl)
                      n112 = Divide(x=w155, y=w152) -> (x/y=→"dLock_in (mV/V)":dbl)
                    }
                  }
                }
                frame "Process" {
                  n113 = Obtain Notifier(notification data type=FALSE) -> (notifier out=w227:refnum<notifier>, error out=w226:errorcluster)  [unwired: 3 in, 1 out]
                  n114 = stacked-sequence {
                    tunnel: w231 -> [w298 _]
                    tunnel: [w288 _] -> w235
                    tunnel: w227 -> [_ w348]
                    tunnel: [_ w346] -> w230
                    tunnel: w226 -> [_ w345]
                    tunnel: [_ w344] -> w228
                    frame #0 {
                      w287 = 1000
                      w272 = "Processing signal" ("Actual Task")
                      n115 = local write "Actual Task"(w272) -> ()
                      n116 = local read "Samples per Channel"() -> (w306:i32)
                      n117 = local read "Rate"() -> (w299:dbl)
                      n118 = local write "Quick Status 5"(w272) -> ()
                      n119 = local read "path"() -> (w274:path)
                      n120 = local read "DC Voltage (V)"() -> (w285:T3)
                      n121 = Multiply(x=1000.0, y="Stabilization Time (s)") -> (x*y=w277:dbl)
                      n122 = Wait (ms)(milliseconds to wait=w277) -> ()  [unwired: 1 out]
                      n123 = call "Lockin_Amplifier_diag_optional.vi"("Reference signal (dialog if empty)"=w274, "Sample Number"=w306, "DC(V)"=w285, "Cutoff Frequency"="Cutoff Frequency (Hz)", "dt"="dt (s)", "Window (s)"="Lock-in Time (s)", "Continous Lock-in"="Continous Lock-in", "Resolution"="Resolution (s)", "averaging time"="Averaging time (s)", "Error In"=w298, "Second"="Second Harmonic", "Sampling Freq"=w299, "tolerance (Deviation)"="Pike Removal (StDev)") -> ("Error Out"=w288:errorcluster, "Signal Spectrum"=w269:cluster{"f0":dbl, "df":dbl, "magnitude":dbl[]}[], "LockIN R (cont/disc)"=→"LockIN R (cont/disc)":waveform(dbl), "MLD & Phase"=w284:T11, "Time Domain Signal"=→"Time Domain Signal":cluster{"xi used":dbl[], "yi":dbl[]}[], "Timetrace_ref"=w271:waveform(dbl)[], "LockIN Theta (cont/disc)"=→"LockIN Theta (cont/disc)":waveform(dbl))  [unwired: 4 in, 4 out]
                      "Signal Spectrum (mVrms/Vdc)" <- w269
                      n124 = Unbundle(w284) -> ("MLD"=w283:dbl, "dMLD"=w282:dbl, "Phase"=→"Phase (deg)":dbl, "dPhase"=→"Phase  dev (deg)":dbl)
                      n125 = Index Array(array=w269, index=1) -> (element=→"Signal Spectrum (mVrms/Vdc) 2":cluster{"f0":dbl, "df":dbl, "magnitude":dbl[]})
                      n126 = local read "Dc mean"() -> (w286:dbl)
                      n127 = flat-sequence {
                        tunnel: w271 -> [w307]
                        tunnel: [w307] -> w270
                        frame #0 {
                          n128 = local write "Oscilloscope 2"(waveform(dbl)[] [{"t0"=timestamp(0 s since 1904-01-01), "dt"=0.001, "Y"=[]}, {"t0"=timestamp(0 s since 1904-01-01), "dt"=0.001, "Y"=[]}] ("Oscilloscope 2")) -> ()
                        }
                      }
                      n129 = Divide(x=w283, y=w286) -> (x/y=w297:dbl)
                      n130 = Divide(x=w282, y=w286) -> (x/y=w296:dbl)
                      n131 = local write "error out"(w288) -> ()
                      n132 = Multiply(x=w296, y=w287) -> (x*y=w293:dbl)
                      n133 = Multiply(x=w297, y=w287) -> (x*y=w294:dbl)
                      n134 = local read "Voltage Divider (10)"() -> (w295:bool)
                      n135 = case shown="False" w295 {
                        tunnel: w294 -> [w310 w315]
                        tunnel: w293 -> [w309 w314]
                        tunnel: [w310 w312] -> w291
                        tunnel: [w309 w311] -> w290
                        frame False {
                        }
                        frame True {
                          w313 = 10
                          n136 = Multiply(x=w315, y=w313) -> (x*y=w312:dbl)
                          n137 = Multiply(x=w314, y=w313) -> (x*y=w311:dbl)
                        }
                      }
                      "MLD (mV/V)" <- w291
                      "dMLD (mV/V)" <- w290
                      n138 = local write "Oscilloscope 2"(w270) -> ()
                    }
                    frame #1 {
                      w321 = "Plotting" ("Actual Task")
                      n139 = local read "Time Resolved"() -> (w330:bool)
                      n140 = case shown="True" w330 {
                        tunnel: [w360 w361] -> w329
                        frame False {
                          n141 = local read "2f Frequency (Hz)"() -> (w360:dbl)
                        }
                        frame True {
                          n142 = local read "Start time"() -> (w365:timestamp)
                          n143 = Get Date/Time In Seconds() -> (seconds since 1Jan1904=w366:timestamp)
                          n144 = Subtract(x=w366, y=w365) -> (x-y=w363:dbl)
                          n145 = To Double Precision Float(number=w363) -> (double precision float=w362:dbl)
                          n146 = Divide(x=w362, y=60.0) -> (x/y=w361:dbl)
                        }
                      }
                      n147 = local read "DC (V)"() -> (w336:cluster{dbl[], dbl[]})
                      n148 = local read "MLD Phase"() -> (w338:cluster{dbl[], dbl[]})
                      n149 = local read "DC Voltage (V) 2"() -> (w334:dbl)
                      n150 = Send Notification(notification=TRUE, notifier=w348, error in (no error)=w345) -> (notifier out=w346:refnum<notifier>, error out=w344:errorcluster)
                      n151 = Unbundle(w336) -> (w335:dbl[])  [unwired: 1 out]
                      n152 = Unbundle(w338) -> (w337:dbl[])  [unwired: 1 out]
                      n153 = local read "MLD (mV/V)"() -> (w343:dbl)
                      n154 = local read "dMLD (mV/V)"() -> (w342:dbl)
                      n155 = local read "Phase  dev (deg)"() -> (w341:dbl)
                      n156 = local read "LD array"() -> (w327:dbl[])
                      n157 = local read "Phase (deg)"() -> (w340:dbl)
                      n158 = Insert Into Array(array=w335, new element=w334) -> (w333:dbl[])  [unwired: 1 in]
                      n159 = local read "Frequency array"() -> (w328:dbl[])
                      n160 = local read "dPhase array"() -> (w351:dbl[])
                      n161 = local read "LD error array"() -> (w349:dbl[])
                      n162 = Insert Into Array(array=w328, new element=w329) -> (w332:dbl[])  [unwired: 1 in]
                      n163 = Insert Into Array(array=w349, new element=w342) -> (w326:dbl[])  [unwired: 1 in]
                      n164 = Insert Into Array(array=w337, new element=w341) -> (w352:dbl[])  [unwired: 1 in]
                      n165 = Insert Into Array(array=w351, new element=w340) -> (w354:dbl[])  [unwired: 1 in]
                      n166 = Insert Into Array(array=w327, new element=w343) -> (w320:dbl[])  [unwired: 1 in]
                      n167 = local write "Frequency array"(w332) -> ()
                      n168 = local write "LD array"(w320) -> ()
                      n169 = Bundle("Frequency array"=w332, "LD array"=w320) -> (w350:T12)  [unwired: 1 in]
                      n170 = local write "Phase array"(w352) -> ()
                      n171 = local write "LD error array"(w326) -> ()
                      n172 = local read "SA 2f (mv/V)"() -> (w318:dbl)
                      n173 = local write "dPhase array"(w354) -> ()
                      n174 = local read "2f Spectrum array"() -> (w316:dbl[])
                      n175 = call "XY error bars_diag.vi"("XY plot"=w350, "Yerror"=w326) -> ("Y error bars"=→"MLD Amplitude (mV/V)":cluster{dbl[], dbl[]})  [unwired: 6 in, 2 out]
                      n176 = Insert Into Array(array=w316, new element=w318) -> (w317:dbl[])  [unwired: 1 in]
                      "2f Spectrum array" <- w317
                      n177 = Array Size(array=w317) -> (size(s)=→"Measured Points":i32)
                      n178 = call <vilib>:"Std Deviation and Variance.vi"("X"=w317) -> ("mean"=w324:dbl, "standard deviation"=→"Delta":dbl)  [unwired: 1 in, 1 out]
                      "Detected Signal (mV/V)" <- w324
                      n179 = Bundle("Frequency array"=w332, w352) -> (w353:cluster{"Frequency array":dbl[], dbl[]})  [unwired: 1 in]
                      n180 = Bundle("Frequency array"=w332, w333) -> (→"DC (V)":cluster{"Frequency array":dbl[], dbl[]})  [unwired: 1 in]
                      n181 = call "XY error bars_diag.vi"("XY plot"=w353, "Yerror"=w354) -> ("Y error bars"=→"MLD Phase":cluster{dbl[], dbl[]})  [unwired: 6 in, 2 out]
                      n182 = local write "Actual Task"(w321) -> ()
                      n183 = local write "Quick Status 5"(w321) -> ()
                      n184 = Greater?(x=w324, y=2.0) -> (0:w325:bool)
                      n185 = case shown="True" w325 {
                        frame False {
                          n186 = local write "Quick Diagnosis"("Not infected" ("Quick Diagnosis")) -> ()
                          n187 = local write "Infected?"(FALSE ("Infected?")) -> ()
                        }
                        frame True {
                          "Infected?" <- TRUE ("Infected?")
                          "Quick Diagnosis" <- "Infected" ("Quick Diagnosis")
                        }
                      }
                    }
                  }
                  n188 = while {
                    tunnel: w231 -> [w261]
                    tunnel: [w253] -> w234
                    tunnel: w227 -> [w260]
                    tunnel: w226 -> [w259]
                    tunnel: [w258] -> w225
                    stop <- w254 stop-if-true
                    n189 = Get Notifier Status(notifier=w260, error in (no error)=w259) -> (current notification=w255:bool, error out=w258:errorcluster)  [unwired: 3 out]
                    n190 = local read "DC Voltage (V) 2"() -> (w257:dbl)
                    n191 = local read "level B"() -> (w249:dbl)
                    n192 = local read "level A"() -> (w250:dbl)
                    n193 = local read "AC?"() -> (w241:bool)
                    n194 = local read "Reference Signal"() -> (w263:tag)
                    n195 = local read "V/div A"() -> (w252:dbl)
                    n196 = local read "LD Signal"() -> (w262:tag)
                    n197 = local read "V/div B"() -> (w251:dbl)
                    n198 = call "fast_scope_diag.vi"("Sensitivity"=T4."-10V..10V", "Reference Signal"=w263, "AC?"=w241, "mean"=w257, "LD Signal"=w262, "V/div"=w252, "error in (no error)"=w261, "Max frequency (Hz)"=200.0, "V/div in B"=w251, "level B"=w249, "Refresh in (s)"=1.0, "level A"=w250) -> ("levelA"=w247:dbl, "levelB"=w246:dbl, "Unbalanced"=w245:bool, "1f Peak (mv/V)"=w239:dbl, "MLD SA (mV/V)"=w238:dbl, "Scale Max"=w242:dbl, "Scale Min"=w244:dbl, "Frequency"=w240:dbl, "Spectrum"=w237:cluster{"f0":dbl, "df":dbl, "magnitude":dbl[]}, "V/div out"=w243:dbl, "Array"=w248:waveform(dbl)[], "error out"=w253:errorcluster)  [unwired: 4 in]
                    n199 = local write "1f SA (mV/V)"(w239) -> ()
                    n200 = local write "Spectrum (mVRMS/Vdc)"(w237) -> ()
                    n201 = local write "Oscilloscope"(w248) -> ()
                    n202 = local write "levelB"(w246) -> ()
                    n203 = local write "levelA"(w247) -> ()
                    n204 = local write "2f Frequency (Hz)"(w240) -> ()
                    n205 = property on="Oscilloscope" class="WFChart (strict)"("YScale.Increment"=w243, "YScale.Maximum"=w242, "YScale.Minimum"=w244) -> ()  [unwired: 2 in, 2 out]
                    n206 = local write "error out"(w253) -> ()
                    n207 = Not(x=w245) -> (.not. x?=w256:bool)
                    n208 = local write "Signal Balance"(w245) -> ()
                    n209 = And(x=w256, y=w255) -> (x .and. y?=w254:bool)
                    n210 = local write "MLD SA (mV/V)"(w238) -> ()
                  }
                  n211 = Merge Errors(w228, w225) -> (w229:errorcluster)
                  n212 = Release Notifier(notifier=w230, error in (no error)=w229) -> ()  [unwired: 1 in, 3 out]
                  n213 = Merge Errors(w235, w234) -> (w233:errorcluster)
                }
                frame "Save" {
                  n214 = local read "dLock_in (mV/V)"() -> (w372:dbl)
                  n215 = case shown="False" "Time Resolved" {
                    tunnel: [w389 w390] -> w368
                    frame False {
                      n216 = local read "2f Frequency (Hz)"() -> (w389:dbl)
                    }
                    frame True {
                      n217 = local read "Start time"() -> (w394:timestamp)
                      n218 = Get Date/Time In Seconds() -> (seconds since 1Jan1904=w395:timestamp)
                      n219 = Subtract(x=w395, y=w394) -> (x-y=w392:dbl)
                      n220 = To Double Precision Float(number=w392) -> (double precision float=w391:dbl)
                      n221 = Divide(x=w391, y=60.0) -> (x/y=w390:dbl)
                    }
                  }
                  n222 = local read "Lock_in (mV/V)"() -> (w373:dbl)
                  n223 = local read "SA 2f (mv/V)"() -> (w374:dbl)
                  n224 = local read "SA 1f (mv/V)"() -> (w375:dbl)
                  n225 = local read "Unbalanced?"() -> (w369:bool)
                  n226 = local read "Phase  dev (deg)"() -> (w384:dbl)
                  n227 = local read "Dc standard deviation"() -> (w382:dbl)
                  n228 = local read "dMLD (mV/V)"() -> (w376:dbl)
                  n229 = local read "MLD (mV/V)"() -> (w377:dbl)
                  n230 = local read "Phase (deg)"() -> (w385:dbl)
                  n231 = local read "Dc mean"() -> (w383:dbl)
                  n232 = Boolean To (0,1)(Boolean=w369) -> (0, 1=w371:i16)
                  n233 = To Double Precision Float(number=w371) -> (double precision float=w370:dbl)
                  n234 = Build Array(w368, w377, w376, w375, w374, w373, w372, w385, w384, w383, w382, w370) -> (w380:dbl[])
                  n235 = global read "Global 1_diag.vi" "Measurement File"() -> (w381:path)
                  n236 = call-poly <vilib>:"Write To Spreadsheet File.vi"("format (%.3f)"="%g", "append to file? (new file:F)"=TRUE, "1D data"=w380, "file path (dialog if empty)"=w381) -> ()  [unwired: 4 in, 1 out]
                  n237 = local read "Last Step?"() -> (w386:bool)
                  n238 = case shown="True" w386 {
                    tunnel: [State_machine_enum."Measure" State_machine_enum."Finished"] -> w387
                    frame False {
                    }
                    frame True {
                    }
                  }
                }
                frame "Finished" {
                  n239 = local read "Last Step?"() -> (w399:bool)
                }
              }
              n240 = local read "Stopped"() -> (w103:bool)
              n241 = Compound Arithmetic op=OR(w105, w104, w103) -> (w102:bool)
              "Actual State" <- w106
            }
          }
          frame #2 {
            # "Terminating"
            n242 = local read "Stopped"() -> (w402:bool)
            n243 = case shown="False" w402 {
              tunnel: w403 -> [w412 _]
              tunnel: [w411 w415] -> w400
              tunnel: w401 -> [w410 w415]
              frame False {
                w404 = "Measurement finished" ("Actual Task")
                n244 = local write "Reset?"(TRUE ("Reset?")) -> ()
                n245 = local write "Actual Task"(w404) -> ()
                n246 = local write "Quick Status 5"(w404) -> ()
                n247 = local read "Motor Voltage (V)"() -> (w405:dbl)
                n248 = local read "Motor Channel"() -> (w408:tag)
                n249 = call "gradual_motorset_diag.vi"("Initial Voltage (V)"=w405, "error in (no error)"=w410, "Steps"=500.0, "Next Voltage (V)"=0.0 ("Numeric"), "Physical Channel"=w408) -> ("error out"=w409:errorcluster)  [unwired: 6 in]
                n250 = Merge Errors(w412, w409) -> (w411:errorcluster)
              }
              frame True {
                n251 = local write "Stopped"(FALSE ("Stopped")) -> ()
              }
            }
            n252 = local write "error out"(w400) -> ()
          }
        }
      }
      frame "stop" {
        n253 = call <vilib>:"Three Button Dialog.vi"("Window Title (\"\")"="Stop Measurement" ("Window Title (\"\")"), "Right Button Text (\"Cancel\")"="Continue" ("Right Button Text (\"Cancel\")"), "Center Button Text (\"No\")"="Pause" ("Right Button Text (\"Cancel\")"), "Left Button Text (\"Yes\")"="Stop and Reset" ("Left Button Text (\"Yes\")"), "message"="Would You like to stop measurement?") -> ("Which Button?"=w419:T9)  [unwired: 6 in]
        n254 = case shown="\"Left Button\", Default" w419 {
          tunnel: w418 -> [w427 w447 w479]
          tunnel: [w426 w446 w479] -> w417
          tunnel: w416 -> [_ w445 w478]
          frame "Left Button", Default {
            # "Stop and reset"
            n255 = local write "Reset?"(TRUE ("Reset?")) -> ()
            n256 = local read "Motor Channel"() -> (w428:tag)
            n257 = global read "Global 1_diag.vi" "Measurement File"() -> (w430:path)
            n258 = call "motor_control_voltage.vi"("Error In"=w427, "Numeric"=0.0, "Physical Channel"=w428) -> ("error out"=w426:errorcluster)  [unwired: 8 in]
            n259 = Not A Number/Path/Refnum?(number/path/refnum=w430) -> (NaN/Path/Refnum?=w431:bool)
            n260 = Empty String/Path?(string/path=w430) -> (empty?=w432:bool)
            n261 = Or(x=w431, y=w432) -> (x .or. y?=w433:bool)
            n262 = case shown="False" w433 {
              tunnel: w430 -> [w434 _]
              frame False {
                n263 = local read "Phase  dev (deg)"() -> (w437:dbl)
                n264 = local read "Dc standard deviation"() -> (w435:dbl)
                n265 = local read "2f Frequency (Hz)"() -> (w441:dbl)
                n266 = local read "dMLD (mV/V)"() -> (w439:dbl)
                n267 = local read "MLD (mV/V)"() -> (w440:dbl)
                n268 = local read "Phase (deg)"() -> (w438:dbl)
                n269 = local read "Dc mean"() -> (w436:dbl)
                n270 = Build Array(w441, w440, w439, w438, w437, w436, w435) -> (w444:dbl[])
                n271 = call-poly <vilib>:"Write To Spreadsheet File.vi"("format (%.3f)"="%g", "append to file? (new file:F)"=TRUE, "1D data"=w444, "file path (dialog if empty)"=w434) -> ()  [unwired: 4 in, 1 out]
              }
              frame True {
              }
            }
          }
          frame "Center Button" {
            # "Pause"
            n272 = local write "Reset?"(FALSE ("Reset?")) -> ()
            n273 = local write "Stopped"(FALSE ("Stopped")) -> ()
            n274 = local write "Actual Task"("Paused" ("Actual Task")) -> ()
            n275 = while {
              tunnel: w447 -> [w469]
              tunnel: [w468] -> w446
              tunnel: w445 -> [w465]
              stop <- w466 stop-if-true
              n276 = local read "Reference Signal"() -> (w473:tag)
              n277 = local read "LD Signal"() -> (w474:tag)
              n278 = Get Queue Status(queue=w465) -> (# elements in queue=w467:i32)  [unwired: 2 in, 7 out]
              n279 = local read "DC Voltage (V) 2"() -> (w464:dbl)
              n280 = local read "AC?"() -> (w463:bool)
              n281 = Greater Than 0?(x=w467) -> (x > 0?=w466:bool)
              n282 = local read "V/div B"() -> (w461:dbl)
              n283 = local read "level A"() -> (w460:dbl)
              n284 = local read "level B"() -> (w459:dbl)
              n285 = local read "V/div A"() -> (w462:dbl)
              n286 = call "fast_scope_diag.vi"("Sensitivity"=T4."-10V..10V", "Reference Signal"=w473, "AC?"=w463, "mean"=w464, "LD Signal"=w474, "V/div"=w462, "error in (no error)"=w469, "Max frequency (Hz)"=200.0, "V/div in B"=w461, "level B"=w459, "Refresh in (s)"=1.0, "level A"=w460) -> ("levelA"=w458:dbl, "levelB"=w457:dbl, "Unbalanced"=w452:bool, "Scale Max"=w455:dbl, "Scale Min"=w454:dbl, "Spectrum"=w451:cluster{"f0":dbl, "df":dbl, "magnitude":dbl[]}, "V/div out"=w453:dbl, "Array"=w456:waveform(dbl)[], "error out"=w468:errorcluster)  [unwired: 4 in, 3 out]
              n287 = local write "levelA"(w458) -> ()
              n288 = local write "levelB"(w457) -> ()
              n289 = local write "Signal Spectrum (mVrms/Vdc) 2"(w451) -> ()
              n290 = local write "Spectrum (mVRMS/Vdc)"(w451) -> ()
              n291 = local write "Signal Balance"(w452) -> ()
              n292 = local write "Oscilloscope"(w456) -> ()
              n293 = property on="Oscilloscope" class="WFChart (strict)"("YScale.Increment"=w453, "YScale.Maximum"=w455, "YScale.Minimum"=w454) -> ()  [unwired: 2 in, 2 out]
            }
          }
          frame "Right Button" {
            # "Continue"
            n294 = Enqueue Element(queue=w478, element=User_buttons_enum."start") -> ()  [unwired: 2 in, 3 out]
            n295 = local write "Stopped"(FALSE ("Stopped")) -> ()
            "Reset?" <- FALSE ("Reset?")
          }
        }
      }
      frame "exit" {
        # "This will stop the consumer loop, thus exit this\nportion of the program."
      }
      frame "New" {
        n296 = call "Create_file_diag.vi"("error in (no error)"=w484) -> ("error out"=w483:errorcluster, "Measurement File out"=w482:path)  [unwired: 9 in]
        n297 = local write "Measurement File"(w482) -> ()
      }
      frame "Scope" {
        w509 = 10123 items=["Finite Samples"=10178, "Continuous Samples"=10123, "Hardware Timed Single Point"=12522]  # sample mode
        w516 = FALSE  # auto cleanup
        n298 = Divide(x=1.0, y="rate") -> (x/y=→"dt":dbl)
        n299 = local read "DC Voltage DAQ"() -> (w486:tag)
        n300 = call <vilib>:"DAQmx Create Task.vi"("auto cleanup"=w516, "error in"=w493) -> ("task out"=w492:refnum<k21>, "error out"=w491:errorcluster)  [unwired: 12 in]
        n301 = local read "Reference Signal"() -> (w518:tag)
        n302 = call-poly <vilib>:"DAQmx Create Virtual Channel.vi"("task in"=w492, "maximum value"=10.0, "minimum value"=-10.0, "physical channels"=w486, "error in"=w491) -> ("task out"=w490:refnum<k21>, "error out"=w489:errorcluster)  [unwired: 9 in]
        n303 = call-poly <vilib>:"DAQmx Create Virtual Channel.vi"("task in"=w490, "maximum value"=10.0, "minimum value"=-10.0, "physical channels"=w518, "error in"=w489) -> ("task out"=w512:refnum<k21>, "error out"=w513:errorcluster)  [unwired: 9 in]
        n304 = local read "LD Signal"() -> (w517:tag)
        n305 = case shown="\"-1V..1V\", Default" "Sensitivity" {
          tunnel: [-1.0 ("maximum value") -1.25 ("maximum value") -2.0 ("maximum value") -2.5 ("maximum value") -4.0 ("maximum value") -5.0 ("maximum value") -10.0 ("maximum value")] -> w507
          tunnel: [1.0 ("maximum value") 1.25 ("maximum value") 2.0 ("maximum value") 2.5 ("maximum value") 4.0 ("maximum value") 5.0 ("maximum value") 10.0 ("maximum value")] -> w506
          frame "-1V..1V", Default {
          }
          frame "-1.25V..1.25V" {
          }
          frame "-2V..2V" {
          }
          frame "-2.5V..2.5V" {
          }
          frame "-4V..4V" {
          }
          frame "-5V..5V" {
          }
          frame "-10V..10V" {
          }
        }
        n306 = call-poly <vilib>:"DAQmx Create Virtual Channel.vi"("task in"=w512, "maximum value"=w506, "minimum value"=w507, "physical channels"=w517, "error in"=w513) -> ("task out"=w510:refnum<k21>, "error out"=w511:errorcluster)  [unwired: 9 in]
        n307 = call-poly <vilib>:"DAQmx Timing.vi"("task/channels in"=w510, "sample mode"=w509, "samples per channel"="samples per channel", "rate"="rate", "error in"=w511) -> ("task out"=w497:refnum<k21>, "error out"=w495:errorcluster)  [unwired: 9 in]
        n308 = property class="DAQmx Channel"(reference=w497, error in=w495, "AI.UsbXferReqCount"=u32 1) -> (reference out=w496:refnum<k21>, error out=w494:errorcluster)
        n309 = while {
          tunnel: [w554] -> w500
          tunnel: w494 -> [w539]
          tunnel: w496 -> [w544]
          tunnel: "samples per channel" -> [w543]
          tunnel: [w541] -> w501
          tunnel: w485 -> [w533]
          stop <- w555 stop-if-true
          n310 = Obtain Queue(element data type=dbl[][] [] ("data")) -> (queue out=w559:refnum<queue>)  [unwired: 4 in, 2 out]
          n311 = while {
            tunnel: w559 -> [w569]
            shift-right: [w563] -> w538
            shift-left: dbl[][] [] ("element data type") -> [w570]
            tunnel: w533 -> [w561]
            i -> [w566]
            stop <- w562 stop-if-true
            n312 = Equal?(x=0, y=w566) -> (x = y?=w564:bool)
            n313 = Dequeue Element(queue=w569) -> (element=w568:dbl[][], error out=w567:errorcluster)  [unwired: 2 in, 2 out]
            n314 = case shown="No Error" w567 {
              tunnel: w568 -> [w582 _]
              tunnel: w570 -> [w603 w686]
              tunnel: w564 -> [w602 _]
              tunnel: [w591 w686] -> w563
              tunnel: [FALSE TRUE] -> w562
              tunnel: w561 -> [w572 _]
              frame No Error {
                n315 = local read "Second Harmonic"() -> (w579:bool)
                n316 = Transpose 2D Array(2D array=w582) -> (transposed array=w581:dbl[][])
                n317 = Index Array(array=w581, index (col)=2) -> (element=w580:dbl[])  [unwired: 1 in]
                n318 = Index Array(array=w581, index (col)=1) -> (element=w586:dbl[])  [unwired: 1 in]
                n319 = Build Array(w586, w580) -> (w584:dbl[][])
                n320 = Transpose 2D Array(2D array=w584) -> (transposed array=w583:dbl[][])
                n321 = Insert Into Array(array=w603, new element=w583) -> (w585:dbl[][])  [unwired: 2 in]
                n322 = local read "dt"() -> (w596:dbl)
                n323 = call "Scopeset_diag.vi"("Ref_MLD measurement"=w583, "V/div in B"="V/div B", "Second"=w579, "AC?"="AC?", "V/div in A"="V/div A", "level B"="level B", "level A"="level A", "dt"=w596) -> ("UP"=w577:bool, "Down"=w578:bool, "V/div out"=w610:dbl, "Ref_MLD_triggered"=w604:dbl[][], "levelB"=→"levelB":dbl, "MLD_mean"=w576:dbl, "Scale Max"=w612:dbl, "Scale Min"=w611:dbl, "levelA"=→"levelA":dbl, "Array"=w571:waveform(dbl)[], "Frequency"=w593:dbl)  [unwired: 7 in, 2 out]
                "Oscilloscope" <- w571
                "Up" <- w577
                "Down" <- w578
                "Oscilloscope 2" <- w571
                n324 = property on="Oscilloscope" class="WFChart (strict)"("YScale.Increment"=w610, "YScale.Maximum"=w612, "YScale.Minimum"=w611) -> ()  [unwired: 2 in, 2 out]
                n325 = local write "2f Frequency (Hz)"(w593) -> ()
                n326 = local write "2f Frequency (Hz)"(w593) -> ()
                n327 = case shown="False" w602 {
                  tunnel: w604 -> [_ w684]
                  tunnel: w585 -> [w683 _]
                  tunnel: [w683 w684] -> w591
                  frame False {
                  }
                  frame True {
                  }
                }
                n328 = Index Array(array=w581, index (col)=0) -> (element=w590:dbl[])  [unwired: 1 in]
                n329 = call-poly <vilib>:"Mean.vi"("X"=w590) -> ("mean"=w574:dbl)  [unwired: 1 out]
                "DC Voltage (V)" <- w574
                n330 = local write "DC Voltage (V) 2"(w574) -> ()
                n331 = Index Array(array=w591, index (col)=1 ("disabled index (col)")) -> (element=w573:dbl[])  [unwired: 1 in]
                n332 = case shown="True" "QuickDiag" {
                  tunnel: w578 -> [_ w620]
                  tunnel: w577 -> [_ w619]
                  tunnel: w576 -> [_ w618]
                  tunnel: w574 -> [_ w617]
                  tunnel: w573 -> [_ w616]
                  tunnel: w571 -> [_ _]
                  tunnel: w572 -> [_ w615]
                  frame False {
                  }
                  frame True {
                    n333 = stacked-sequence {
                      tunnel: w620 -> [_ _ w644 _]
                      tunnel: w619 -> [_ _ w643 _]
                      tunnel: w618 -> [_ _ w640 _]
                      tunnel: w617 -> [w624 w634 _ _]
                      tunnel: w616 -> [_ w633 _ _]
                      tunnel: w615 -> [_ _ _ _]
                      frame #0 {
                        n334 = local write "Quick Status 5"("Checking LASER" ("Quick Status 5")) -> ()
                        n335 = Greater?(x=w624, y=1.0) -> (0:w621:bool)
                        n336 = case shown="True" w621 {
                          frame False {
                            n337 = local write "Laser Intensity"("Laser Intensity: Too low" ("Laser Intensity")) -> ()
                            n338 = local write "Laser Intensity"(FALSE ("Laser Intensity")) -> ()
                          }
                          frame True {
                            "Laser Intensity" <- TRUE ("Laser Intensity")
                            "Laser Intensity" <- "Laser Intensity: OK" ("Laser Intensity")
                          }
                        }
                      }
                      frame #1 {
                        n339 = call <vilib>:"Std Deviation and Variance.vi"("X"=w633) -> ("standard deviation"=w632:dbl)  [unwired: 1 in, 2 out]
                        n340 = Divide(x=w632, y=w634) -> (x/y=w631:dbl)
                        "x/y" <- w631
                        n341 = Less?(x=w631, y=0.05) -> (x < y?=w629:bool)
                        n342 = case shown="True" w629 {
                          frame False {
                            n343 = local write "Laser Noise"("Laser Noise: Too High" ("Laser Noise")) -> ()
                            n344 = local write "Laser Noise"(FALSE ("Laser Noise")) -> ()
                          }
                          frame True {
                            "Laser Noise" <- TRUE ("Laser Noise")
                            "Laser Noise" <- "Laser Noise: OK" ("Laser Noise")
                          }
                        }
                      }
                      frame #2 {
                        n345 = Absolute Value(x=w640) -> (abs(x)=w642:dbl)
                        n346 = Less?(x=w642, y=0.2) -> (x < y?=w639:bool)
                        n347 = case shown="True" w639 {
                          frame False {
                            n348 = local write "Signal Balance"(FALSE ("Signal Balance")) -> ()
                            "Signal Balance" <- "Signal Balance : Unbalanced" ("Signal Balance")
                          }
                          frame True {
                            n349 = local write "Signal Balance"("Signal Balance: OK" ("Signal Balance")) -> ()
                            "Signal Balance" <- TRUE ("Signal Balance")
                          }
                        }
                        "Down 2" <- w644
                        "Up 2" <- w643
                      }
                      frame #3 {
                        n350 = local read "Laser Intensity"() -> (w650:bool)
                        n351 = local read "Laser Noise"() -> (w651:bool)
                        n352 = local read "Signal Balance"() -> (w652:bool)
                        n353 = Compound Arithmetic op=AND(w650, w651, w652) -> (w649:bool)
                        n354 = case shown="True" w649 {
                          frame False {
                          }
                          frame True {
                            n355 = stacked-sequence {
                              frame #0 {
                                n356 = property on="Constant Motor Voltage" class="DigNum (strict)"("Val(Sgnl)"=1.0 ("Value (Signaling)")) -> ()  [unwired: 2 in, 2 out]
                                n357 = local write "Quick Status 5"("LASER OK, Motor ON" ("Quick Status 5")) -> ()
                              }
                              frame #1 {
                                n358 = local read "2f Frequency (Hz)"() -> (w659:T3)
                                n359 = Greater?(x=w659, y=T3 18.0) -> (0:w656:bool)
                                n360 = Less?(x=w659, y=T3 21.0) -> (x < y?=w655:bool)
                                n361 = And(x=w656, y=w655) -> (x .and. y?=w657:bool)
                                n362 = case shown="True" w657 {
                                frame False {
                                n363 = local write "Motor"("Motor:...  " ("Motor")) -> ()
                                n364 = local write "Motor"(FALSE ("Motor")) -> ()
                                }
                                frame True {
                                n365 = local write "QuickDiag"(FALSE ("QuickDiag")) -> ()
                                n366 = local write "Ready?"(TRUE ("Ready?")) -> ()
                                n367 = property on="Measure" class="Bool"("DisabledEnum"=T8."Enabled" ("Disabled")) -> ()  [unwired: 2 in, 2 out]
                                "Motor" <- TRUE ("Motor")
                                "Motor" <- "Motor: OK" ("Motor")
                                }
                                }
                              }
                            }
                          }
                        }
                      }
                    }
                  }
                }
                n368 = Bundle By Name("Y"=w573, "dt"=w596) -> (w589:waveform(dbl))  [unwired: 1 in]
                n369 = case shown="False" "Lock In" {
                  tunnel: w574 -> [_ w668]
                  frame False {
                  }
                  frame True {
                    n370 = local read "Lock-in-Amplifier VISA"() -> (w672:refnum<visa-resource-name>)
                    n371 = call "Lock_in_single_meas.vi"("Lock-in-Amplifier VISA"=w672) -> ("Lockin_ampl"=w670:dbl, "Freq"=→"Lockin_freq":dbl)  [unwired: 7 in, 2 out]
                    n372 = xnode "LIA calc"("X1"=w670, "X2"=w668) -> ("Result"=→"MLD LIA (mV/V)":dbl)  [unwired: 1 in, 1 out]
                  }
                }
                n373 = call "Fast_spectrum_analyzer_diag.vi"("mean"=w574, "Waveform"=w589, "Frequency"=w593) -> ("error out"=w601:errorcluster, "MLD SA (mV/V)"=w595:dbl, "Spectrum (mV/V)"=→"Spectrum (mVRMS/Vdc)":cluster{"f0":dbl, "df":dbl, "magnitude":dbl[]}, "1f Peak (mv/V)"=w594:dbl)  [unwired: 5 in]
                n374 = local write "MLD SA (mV/V)"(w595) -> ()
                n375 = local write "1f SA (mV/V)"(w594) -> ()
                n376 = local write "error out"(w601) -> ()
              }
              frame Error {
              }
            }
          }
          n377 = while {
            tunnel: [w702] -> w541
            shift-right: [w687] -> w542
            shift-left: w539 -> [w703]
            tunnel: [w699] -> _
            tunnel: w559 -> [w698]
            tunnel: [w696] -> w558
            tunnel: w544 -> [w695]
            tunnel: w543 -> [w694]
            tunnel: ["stop"] -> w534
            i -> [w693]
            stop <- w699 stop-if-true
            w700 = 10.0  # timeout (s)
            n378 = Subtract(x="Refresh in (s)", y=i8 2) -> (x-y=w691:i8)
            n379 = Less?(x=w691, y=w693) -> (x < y?=w692:bool)
            n380 = call-poly <vilib>:"DAQmx Read.vi"("task/channels in"=w695, "number of samples per channel"=w694, "timeout"=w700, "error in"=w703) -> ("task out"=w702:refnum<k21>, "data"=w697:dbl[][], "error out"=w687:errorcluster)  [unwired: 9 in]
            n381 = Unbundle By Name(w687) -> ("status"=w701:bool)
            n382 = local write "error out"(w687) -> ()
            n383 = Enqueue Element(queue=w698, element=w697) -> (queue out=w696:refnum<queue>)  [unwired: 2 in, 2 out]
            n384 = Compound Arithmetic op=OR(w701, "stop", w692) -> (w699:bool)
            "result" <- w699
          }
          n385 = local read "Continous Lock-in"() -> (w535:bool)
          n386 = Merge Errors(w542) -> (w553:errorcluster)
          n387 = case shown="True" w534 {
            frame False {
            }
            frame True {
              n388 = local write "stop"(FALSE ("stop")) -> ()
            }
          }
          n389 = Release Queue(queue=w558, error in (no error)=w553) -> (error out=w554:errorcluster)  [unwired: 1 in, 2 out]
          n390 = local read "DC Voltage (V) 2"() -> (w536:dbl)
          n391 = local read "Refresh in (s)"() -> (w549:i8)
          n392 = Array Size(array=w538) -> (size(s)=w547:i32[])
          n393 = Transpose 2D Array(2D array=w538) -> (transposed array=w537:dbl[][])
          n394 = Index Array(array=w547, index=0) -> (element=w548:i32)
          n395 = local read "rate"() -> (w551:dbl)
          n396 = local read "dt"() -> (w552:dbl)
          n397 = local read "Second Harmonic"() -> (w546:bool)
          n398 = call "Lockin_Amplifier_diag_fast.vi"("Refresh in (s)"=w549, "dt"=w552, "mean"=w536, "Continous Lock-in"=w535, "Ref_MLD measurement"=w537, "Second"=w546, "Number of samples"=w548, "Sampling frequency"=w551) -> ("Result 2"=w540:dbl, "Result"=→"dLD_RMS":dbl)  [unwired: 6 in]
          n399 = local write "MLD Sim. LIA (mV/V)"(w540) -> ()
          n400 = Compound Arithmetic op=OR(w534, w554) -> (w555:bool)
        }
        n401 = call <vilib>:"DAQmx Clear Task.vi"("task in"=w501, "error in"=w500) -> ("error out"=w499:errorcluster)  [unwired: 13 in]
      }
    }
    n402 = Unbundle By Name(w14) -> ("status"=w13:bool)
    n403 = Or(x=w13, y=w12) -> (x .or. y?=w11:bool)
  }
  n404 = while {
    shift-right: [w706] -> w6
    shift-left: w9 -> [w709]
    tunnel: w2 -> [w710]
    tunnel: [w704] -> w7
    stop <- w707 stop-if-true
    # "This loop is the producer loop."
    n405 = event shown="[5] \"Start Scope\": Value Change" {
      selector: _ -> [_ _ _ _ _ _ _ _ _ _ _ _ _ _]
      dyn-events: _ -> [_ _ _ _ _ _ _ _ _ _ _ _ _ _]
      timeout: _ -> [_ _ _ w729 _ _ _ _ _ _ _ _ _ _]
      tunnel: w710 -> [w715 w720 w727 w731 w740 w746 _ _ _ _ _ _ _ w822]
      tunnel: w709 -> [w714 w721 w725 w734 w739 w745 w752 _ _ _ _ _ w815 w821]
      tunnel: [w713 w718 w724 w733 w737 w743 w749 _ _ _ _ _ w815 w820] -> w706
      tunnel: [_ _ _ "EXIT" _ _ _ _ _ _ _ _ _ _] -> w708
      tunnel: [w712 w719 w726 w732 w738 w744 _ _ _ _ _ _ _ w819] -> w704
      tunnel: [_ _ _ w729 _ _ _ _ _ _ _ _ _ _] -> _
      event "Start Measurement Button": Value Change {
        n406 = event-data() -> ()  [unwired: 1 in, 1 out]
        n407 = Enqueue Element(queue=w715, element=User_buttons_enum."start", error in (no error)=w714) -> (queue out=w712:refnum<queue>, error out=w713:errorcluster)  [unwired: 1 in, 1 out]
      }
      event "Stop Measurement": Value Change {
        n408 = event-data() -> ()  [unwired: 1 in, 1 out]
        n409 = Enqueue Element(queue=w720, element=User_buttons_enum."stop", error in (no error)=w721) -> (queue out=w719:refnum<queue>, error out=w718:errorcluster)  [unwired: 1 in, 1 out]
        "Stopped" <- TRUE
      }
      event "Measure": Value Change {
        n410 = event-data() -> ()  [unwired: 1 in, 3 out]
        n411 = local write "stop"(TRUE ("stop")) -> ()
        n412 = local write "QuickDiag"(FALSE ("QuickDiag")) -> ()
        n413 = Enqueue Element(queue=w727, element=User_buttons_enum."start", error in (no error)=w725) -> (queue out=w726:refnum<queue>, error out=w724:errorcluster)  [unwired: 1 in, 1 out]
      }
      event "EXIT": Value Change {
        n414 = event-data() -> ()  [unwired: 1 in, 1 out]
        n415 = Enqueue Element(queue=w731, element=User_buttons_enum."exit", error in (no error)=w734) -> (queue out=w732:refnum<queue>, error out=w733:errorcluster)  [unwired: 1 in, 1 out]
      }
      event "New File": Value Change {
        n416 = event-data() -> ()  [unwired: 1 in, 1 out]
        n417 = Enqueue Element(queue=w740, element=User_buttons_enum."New", error in (no error)=w739) -> (queue out=w738:refnum<queue>, error out=w737:errorcluster)  [unwired: 1 in, 1 out]
      }
      event "Start Scope": Value Change {
        n418 = event-data() -> ()  [unwired: 1 in, 1 out]
        n419 = Enqueue Element(queue=w746, element=User_buttons_enum."Scope", error in (no error)=w745) -> (queue out=w744:refnum<queue>, error out=w743:errorcluster)  [unwired: 1 in, 1 out]
        n420 = local write "QuickDiag"(FALSE ("QuickDiag")) -> ()
      }
      event "Constant Motor Voltage": Value Change {
        n421 = event-data() -> ()  [unwired: 1 in, 1 out]
        n422 = local read "Motor Voltage (V)"() -> (w751:dbl)
        n423 = local read "Motor Channel"() -> (w754:tag)
        n424 = call "gradual_motorset_diag.vi"("Initial Voltage (V)"=w751, "error in (no error)"=w752, "Steps"=100.0, "Next Voltage (V)"="Constant Motor Voltage", "Physical Channel"=w754) -> ("error out"=w750:errorcluster)  [unwired: 6 in]
        n425 = case shown="Error" w750 {
          selector: w750 -> [w756 w757]
          tunnel: [w756 w757] -> w749
          tunnel: "Constant Motor Voltage" -> [w755 _]
          tunnel: [w755 0.0 ("Constant Motor Voltage")] -> w747
          frame No Error {
          }
          frame Error {
          }
        }
        n426 = local write "Motor Voltage (V)"(w747) -> ()
      }
      event "Convert dT": Value Change {
        n427 = event-data() -> ()  [unwired: 1 in, 1 out]
        n428 = local read "dT/T (%)"() -> (w767:dbl)
        n429 = local read "Dilution"() -> (w761:dbl)
        n430 = Multiply(x=w767, y=1200.0) -> (x*y=w768:dbl)
        n431 = Divide(x=w767, y=0.0012) -> (x/y=w760:dbl)
        n432 = Multiply(x=w761, y=w760) -> (x*y=w759:dbl)
        n433 = local write "Undiluted cc.\n (ng/ml)"(w759) -> ()
        n434 = local write "MLD (mV/V)"(w768) -> ()
        n435 = Multiply(x=w759, y=2.0) -> (x*y=w764:dbl)
        n436 = Multiply(x=w764, y=2e-05) -> (x*y=w762:dbl)
        n437 = local write "Undiluted \nParasitemia (%)"(w762) -> ()
        n438 = local write "Parasites/ul\nof Blood"(w764) -> ()
      }
      event "Convert mld": Value Change {
        n439 = event-data() -> ()  [unwired: 1 in, 1 out]
        n440 = local read "MLD (mV/V)"() -> (w772:dbl)
        n441 = local read "Dilution"() -> (w774:dbl)
        n442 = Divide(x=w772, y=1200.0) -> (x/y=w771:dbl)
        n443 = Divide(x=w771, y=0.0012) -> (x/y=w773:dbl)
        n444 = Multiply(x=w774, y=w773) -> (x*y=w770:dbl)
        n445 = local write "Undiluted cc.\n (ng/ml)"(w770) -> ()
        n446 = local write "dT/T (%)"(w771) -> ()
        n447 = Multiply(x=w770, y=2.0) -> (x*y=w777:dbl)
        n448 = Multiply(x=w777, y=2e-05) -> (x*y=w775:dbl)
        n449 = local write "Undiluted \nParasitemia (%)"(w775) -> ()
        n450 = local write "Parasites/ul\nof Blood"(w777) -> ()
      }
      event "Convert cc": Value Change {
        n451 = event-data() -> ()  [unwired: 1 in, 1 out]
        n452 = local read "Undiluted cc.\n (ng/ml)"() -> (w781:dbl)
        n453 = local read "Dilution"() -> (w787:dbl)
        n454 = Divide(x=w781, y=w787) -> (x/y=w786:dbl)
        n455 = Multiply(x=w781, y=2.0) -> (x*y=w788:dbl)
        n456 = Multiply(x=0.0012 ("y"), y=w786) -> (x*y=w784:dbl)
        n457 = local write "Parasites/ul\nof Blood"(w788) -> ()
        n458 = local write "dT/T (%)"(w784) -> ()
        n459 = Multiply(x=w788, y=2e-05) -> (x*y=w791:dbl)
        n460 = local write "Undiluted \nParasitemia (%)"(w791) -> ()
        n461 = Multiply(x=1200.0 ("y"), y=w784) -> (x*y=w782:dbl)
        n462 = local write "MLD (mV/V)"(w782) -> ()
      }
      event "Convert parasitemia": Value Change {
        n463 = event-data() -> ()  [unwired: 1 in, 1 out]
        n464 = local read "Undiluted \nParasitemia (%)"() -> (w798:dbl)
        n465 = Divide(x=w798, y=2e-05) -> (x/y=w801:dbl)
        n466 = local read "Dilution"() -> (w802:dbl)
        n467 = Divide(x=w801, y=2.0) -> (x/y=w793:dbl)
        n468 = Divide(x=w793, y=w802) -> (x/y=w792:dbl)
        n469 = Multiply(x=0.0012 ("y"), y=w792) -> (x*y=w796:dbl)
        n470 = local write "dT/T (%)"(w796) -> ()
        n471 = local write "Undiluted cc.\n (ng/ml)"(w793) -> ()
        n472 = local write "Parasites/ul\nof Blood"(w801) -> ()
        n473 = Multiply(x=1200.0 ("y"), y=w796) -> (x*y=w794:dbl)
        n474 = local write "MLD (mV/V)"(w794) -> ()
      }
      event "Convert parasiteno": Value Change {
        n475 = event-data() -> ()  [unwired: 1 in, 1 out]
        n476 = local read "Parasites/ul\nof Blood"() -> (w805:dbl)
        n477 = Multiply(x=w805, y=2e-05) -> (x*y=w813:dbl)
        n478 = local read "Dilution"() -> (w812:dbl)
        n479 = Divide(x=w805, y=2.0) -> (x/y=w804:dbl)
        n480 = local write "Undiluted \nParasitemia (%)"(w813) -> ()
        n481 = Divide(x=w804, y=w812) -> (x/y=w803:dbl)
        n482 = Multiply(x=0.0012 ("y"), y=w803) -> (x*y=w808:dbl)
        n483 = local write "dT/T (%)"(w808) -> ()
        n484 = local write "Undiluted cc.\n (ng/ml)"(w804) -> ()
        n485 = Multiply(x=1200.0 ("y"), y=w808) -> (x*y=w806:dbl)
        n486 = local write "MLD (mV/V)"(w806) -> ()
      }
      event "Timer Start": Value Change {
        n487 = event-data() -> ()  [unwired: 1 in, 3 out]
        n488 = Get Date/Time In Seconds() -> (seconds since 1Jan1904=w814:timestamp)
        n489 = local write "Start time"(w814) -> ()
      }
      event "Run Quick Diagnostics": Value Change {
        n490 = event-data() -> ()  [unwired: 1 in, 3 out]
        n491 = local write "QuickDiag"(TRUE ("QuickDiag")) -> ()
        n492 = Enqueue Element(queue=w822, element=User_buttons_enum."Scope", error in (no error)=w821) -> (queue out=w819:refnum<queue>, error out=w820:errorcluster)  [unwired: 1 in, 1 out]
        n493 = property on="Measure" class="Bool"("DisabledEnum"=T8."Disabled and Grayed Out" ("Disabled")) -> ()  [unwired: 2 in, 2 out]
        "Ready?" <- FALSE ("Ready?")
      }
    }
    n494 = Unbundle By Name(w706) -> ("status"=w705:bool)
    n495 = Or(x=w705, y=w708) -> (x .or. y?=w707:bool)
  }
  n496 = local read "Sensitivity"() -> (w1:T4)
  n497 = case shown="\"-1V..1V\", Default" w1 {
    tunnel: [-1.0 ("maximum value") -1.25 ("maximum value") -2.0 ("maximum value") -2.5 ("maximum value") -4.0 ("maximum value") -5.0 ("maximum value") -10.0 ("maximum value")] -> _
    tunnel: [1.0 ("maximum value") 1.25 ("maximum value") 2.0 ("maximum value") 2.5 ("maximum value") 4.0 ("maximum value") 5.0 ("maximum value") 10.0 ("maximum value")] -> _
    frame "-1V..1V", Default {
    }
    frame "-1.25V..1.25V" {
    }
    frame "-2V..2V" {
    }
    frame "-2.5V..2.5V" {
    }
    frame "-4V..4V" {
    }
    frame "-5V..5V" {
    }
    frame "-10V..10V" {
    }
  }
  n498 = Merge Errors(w6, w5) -> (w4:errorcluster)
  n499 = Release Queue(queue=w7, error in (no error)=w4) -> ()  [unwired: 1 in, 3 out]
